vi "ImagingCore(HS).vi"(5 "BioMAP file path":path=path "", 7 "Params.":variant, 8 "error in (no error)":errorcluster, 9 "Dynamic Params queue":refnum<queue>, 10 "Quit_UserEvent":refnum<user-event>, 11 "ControlQueueRef":variant) -> (0 "error out":errorcluster, 2 "Output":variant)   [LabVIEW 2014]
uses:
  Apps_static/ScanParams_SingleLine.ctl
  Files/BinaryHeader.ctl
  ControlDef/QueueRefs.ctl
  ControlDef/LaserCtrl_Method.ctl
  ControlDef/States-AToF.ctl
  <instrlib>/GenericDAQ/VI/GenericDAQ_Ctrl_Queue.ctl
  <instrlib>/GenericDAQ/VI/GenericDAQ_State.ctl
  <instrlib>/ESP300/Public/Data/ESP300_State.ctl
  <instrlib>/DG535/Command/DG535_States.ctl
  Hardware/BNC(QuantumComposers)/BNC_States.ctl
  Hardware/FemtoLaser(Legacy)/Laser_Status.ctl
  Hardware/DAQmx(Legacy)/DAQmx_Status.ctl
  ControlDef/Signal.ctl
  ProcessMethods/SignalAverager/ProcessStates.ctl
  Files/WriterState.ctl
  <instrlib>/GenericDAQ/VI/GenericDAQ_Signal.ctl
  Hardware/EPM2000(Legacy)/EPM2K_Status.ctl
  ControlDef/SampleRateSelector.ctl
  ImagingMS/DirectImaging_State.ctl
  ImagingMS/Imaging_Params.ctl
  ProcessMethods/BioMapConversion/BioMAPWriterCoreParams.ctl
  ProcessMethods/Binning/BinType.ctl
  <vilib>/Utility/error.llb/DialogType.ctl
  <vilib>/Utility/miscctls.llb/LVRowAndColumnTypeDef.ctl
  <vilib>/picture/picture.llb/imagedata.ctl
  <vilib>/regexp/Match Regular Expression.xnode
  <instrlib>/ESP300/ESP300.lvlib
  <instrlib>/DG535/SRS_DG535_Lib.lvlib
  <userlib>/Utility/ErrorLog_lib.lvlib
  <instrlib>/GenericDAQ/GenericDAQ.lvlib
panel:
  out "Numeric":i32
  out "elements":i32[](array[numeric])
  out "segment #":i32
  out "EOL interval":dbl format="%#.6f"
  out "discarded ct":i32
  out "Flag":T1(ring)
  out "line time":dbl
  out "EOL time":dbl format="%_19f"
  out "line start time":dbl format="%_19f"
  in  "Full Image":bool
  out "flushing time":dbl
  in  "Contrast":cluster{dbl, dbl}(slide)={0.0, 255.0} scale=0.0..255.0
  in  "MaxiMass":dbl=300.0 format="%#_13g"
  in  "Binning":bool
  out "Information":string
  in  "AutoScaleZ":bool
  in  "SaveImage":bool
  in  "Color Scheme":T2(ring)=enum."Rainbow"
  out "#SOL":i32
  out "#EOL":i32
  out "remaining lines":i32
  out "State":T3(ring)
  out "Line# (Y_Img)":i32
  in  "Cancel":bool
  in  "Close/Quit":bool
  in  "Peaks of Interest (32 max)":string[][](table)=[["300", "300"], ["58", ".45"], ["92", ".45"], ["114", ".45"]]
  out "# average":i32
  in  "Start":bool
  out "ImagePreview":dbl[][](graph)
  in  "PeakOI #":i32 min=0 step=1
  out "MS (Raw)":cluster{"m/z_Array":dbl[], sgl[]}(graph)
  out "Iteration":i32
  out "Export File Path":path caption="Filename"
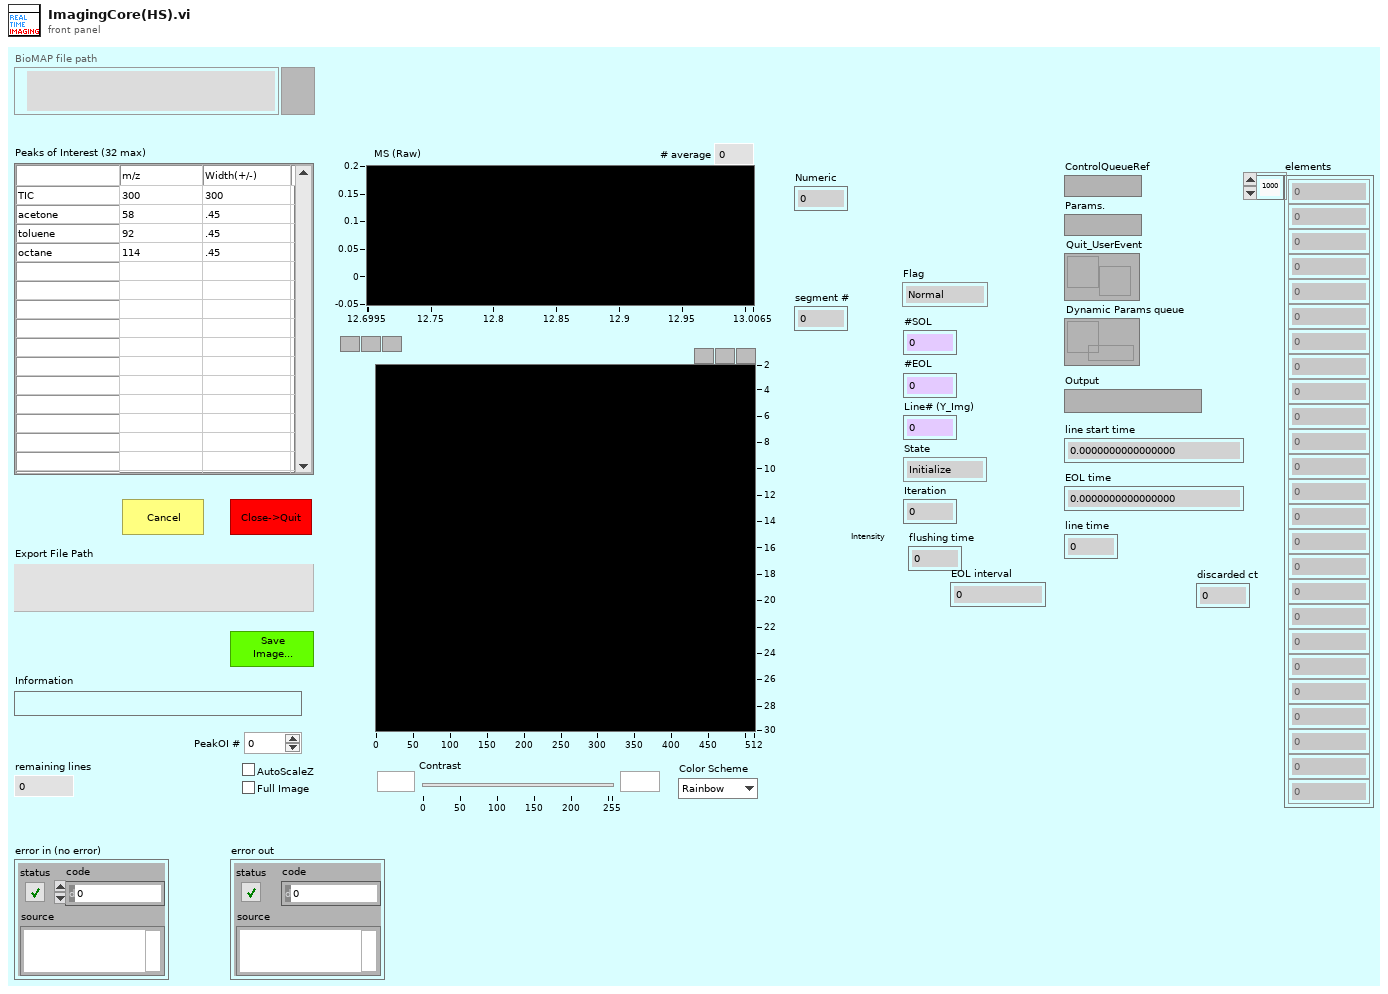
[diagram p1: front panel]
types:
  T1 = enum16{"Normal", "LineStart", "LineEnd", "FrameStart", "FrameEnd", "Reserved1", "Reserved2"}
  T2 = enum16{"Greyscale", "Rainbow", "Jet", "Rainbow_Wh", "Banded", "Seis", "InvertSeis", "Jaisnd", "TBD1"}
  T3 = enum16{"Initialize", "Open", "PrepScanParams", "WaitData", "Flush", "ScanResult", "CheckEndCondition", "Close", "Quit", "Refresh_Image", "Refresh_Profile", "Refresh_Spectra", "Refresh_RawSpectrum", "SaveMiddleFile", "Save_Image", "SetPeakOI"}
  T4 = enum8{"Enabled", "Disabled", "Disabled and Grayed Out"}
  T5 = typedef "QueueRefs.ctl" = cluster{"LaserCtrlMethod":T6, "Apps":refnum<queue>, "MainDAQCoreQueue":refnum<queue>, "Micos":refnum<queue>, "ESP300":refnum<queue>, "SMC100":refnum<queue>, "SRS DG535":refnum<queue>, "BNC":refnum<queue>, "SDG_ii":refnum<queue>, "NI-USB_DAQmx":refnum<queue>, "ProcCore_CtrlQueue":refnum<queue>, "WriterCtrl":refnum<queue>, "WriterSIG":refnum<queue>, "Feedback":refnum<queue>, "EPM2000":refnum<queue>, "InfoRef":refnum<vi>, "AppsLock":T7, "ProcCore_SignalBuffer":refnum<queue>}
  T6 = typedef "LaserCtrl_Method.ctl" = enum16{"SRS_DG535", "BNC", "SDG_II", "GenericDAQ_Sim"}
  T7 = typedef "Semaphore RefNum" = refnum<k1>
  T8 = typedef "BioMAPWriterCoreParams.ctl" = cluster{"File Header":T9, "mzCali.":dbl[], "m/z_Array":dbl[], "SampleRate":T10, "TrigDelay":dbl, "file refnum":refnum<file>, "file path":path, "PeakOI":cluster{"m/z":dbl, "Width(+/-)":dbl}[], "Binning":cluster{"Enable":bool, "BinType":T11, "BinWidth":dbl, "Maximum":dbl, "Minimum":dbl}}
  T9 = typedef "BinaryHeader.ctl" = cluster{"Start Position":dbl[], "StepWidth":dbl[], "Dimension":i32[], "SpecLength":i32}
  T10 = typedef "SampleRateSelector.ctl" = dbl
  T11 = typedef "BinType.ctl" = enum16{"ByTime", "ByScreen", "ByMass", "ToUnitMass"}
  T12 = typedef "Imaging_Params.ctl" = cluster{"File Header":T9, "ScanSpeed":dbl, "HighSpeed":dbl, "SampleRate":T10, "Rep.Rate (Hz)":dbl, "TrigDelay":dbl, "mzCali":dbl[], "KeepStill(ms)":u32, "SaveRaw":bool, "MultiRec":bool}
  T13 = typedef "DirectImaging_State.ctl" = cluster{"State":enum16{"Initialize", "Open", "PrepScanParams", "WaitData", "Flush", "ScanResult", "CheckEndCondition", "Close", "Quit", "Refresh_Image", "Refresh_Profile", "Refresh_Spectra", "Refresh_RawSpectrum", "SaveMiddleFile", "Save_Image", "SetPeakOI"}, "Para.":variant}
  T14 = cluster{"Save?":bool, "File Header":T9, "Scan#":i32, "ControlRefs":T5, "HighSpeed":dbl, "ScanSpeed":dbl, "SampleRate":T10, "mzCali.":dbl[], "TrigDelay":dbl, "InfoBarRef.":refnum<vi>, "MultiRec Mode":bool, "EOL_cts":i32, "SOL_cts":i32}
  T15 = typedef "LVRowAndColumnTypeDef.ctl" = cluster{"Row":i32, "Column":i32}
  T16 = typedef "DialogType.ctl" = u16
  T17 = typedef "GenericDAQ.lvlib/GenericDAQ_Signal.ctl" = cluster{"tickcount":u32, "Signal":sgl[], "SecondaryData":dbl[], "Flag":enum16{"Normal", "LineStart", "LineEnd", "FrameStart", "FrameEnd", "Reserved1", "Reserved2"}, "Segment#":i32}
  T18 = enum16{"open", "replace", "create", "open or create", "replace or create", "replace or create with confirmation"}
  T19 = typedef "Signal.ctl" = cluster{"Command":T20, "Params":variant}
  T20 = typedef "ProcessStates.ctl" = enum16{"Initialize", "Normal", "Display", "Write2Buffer", "CalcMzArray", "StartSave", "StopSave", "ConfigChanged", "EndOfLine", "SetFilterParams", "SetGraphsEnable", "SetAcquisitionParams", "ChangeDisplayIncrement", "ChangeRepRate", "SetWriterRef", "Quit", "StartOfLine"}
  T21 = typedef "GenericDAQ.lvlib/GenericDAQ_Ctrl_Queue.ctl" = cluster{"GenericDAQ State":T22, "Variant":variant}
  T22 = typedef "GenericDAQ.lvlib/GenericDAQ_State.ctl" = enum16{"Enumerate", "Open", "Close", "CloseAll", "Reset", "Quit", "==Settings==", "SetAcquisition_", "SetChannels_", "SetTrigger_", "SetAnalogTrigDetector_", "SetSegment#_", "SetAll_AcquChTrig_", "fConfigurate", "fStart", "GetStatus", "_WaitForDone/Idle", "_GetData", "GetAcquisition", "GetChannels", "GetTrigger", "GetAll_AcquChTrig", "Abort", "==Messaging==", "_PushDataOut", "GetStat_", "GetConfig_", "==ModeSetup==", "SetSignalBuffer_", "SetMode_", "SetSecondaryDataRef._", "SetDynamicBuffer_", "==AnalogOut==", "GetChannelCount_AO", "fStart_AO", "SetChEnable_AO", "SetConfig_AO", "SetFuncData_AO", "SetOffset_AO_", "SetMasterNode_AO", "SetStates_AO", "SetSymetry_AO", "SetTriggerSource_AO", "==Trigger==", "ManualTrigger", "===Sync===", "LineStart", "LineEnd", "FrameStart", "FrameEnd", "EOL_PassThrough", "SOL_PassThrough"}
  T23 = typedef "ScanParams_SingleLine.ctl" = cluster{"Line Start":dbl[], "Line End":dbl[], "HighSpeed":dbl, "ScanSpeed":dbl, "KeepStill(ms)":u32, "SecendaryParams":variant}
  T24 = typedef "imagedata.ctl" = cluster{"image type":i32, "image depth":i32, "image":u8[], "mask":u8[], "colors":u32[], "Rectangle":cluster{"left":i16, "top":i16, "right":i16, "bottom":i16}}
  T25 = cluster{"Rows Per Strip":i32, "Photometric":i32, "Compression Type":i32}
  T26 = cluster{"queue out":refnum<queue>, "queue out":refnum<queue>}
  T27 = typedef "IMAQ Image.ctl" = refnum<image>
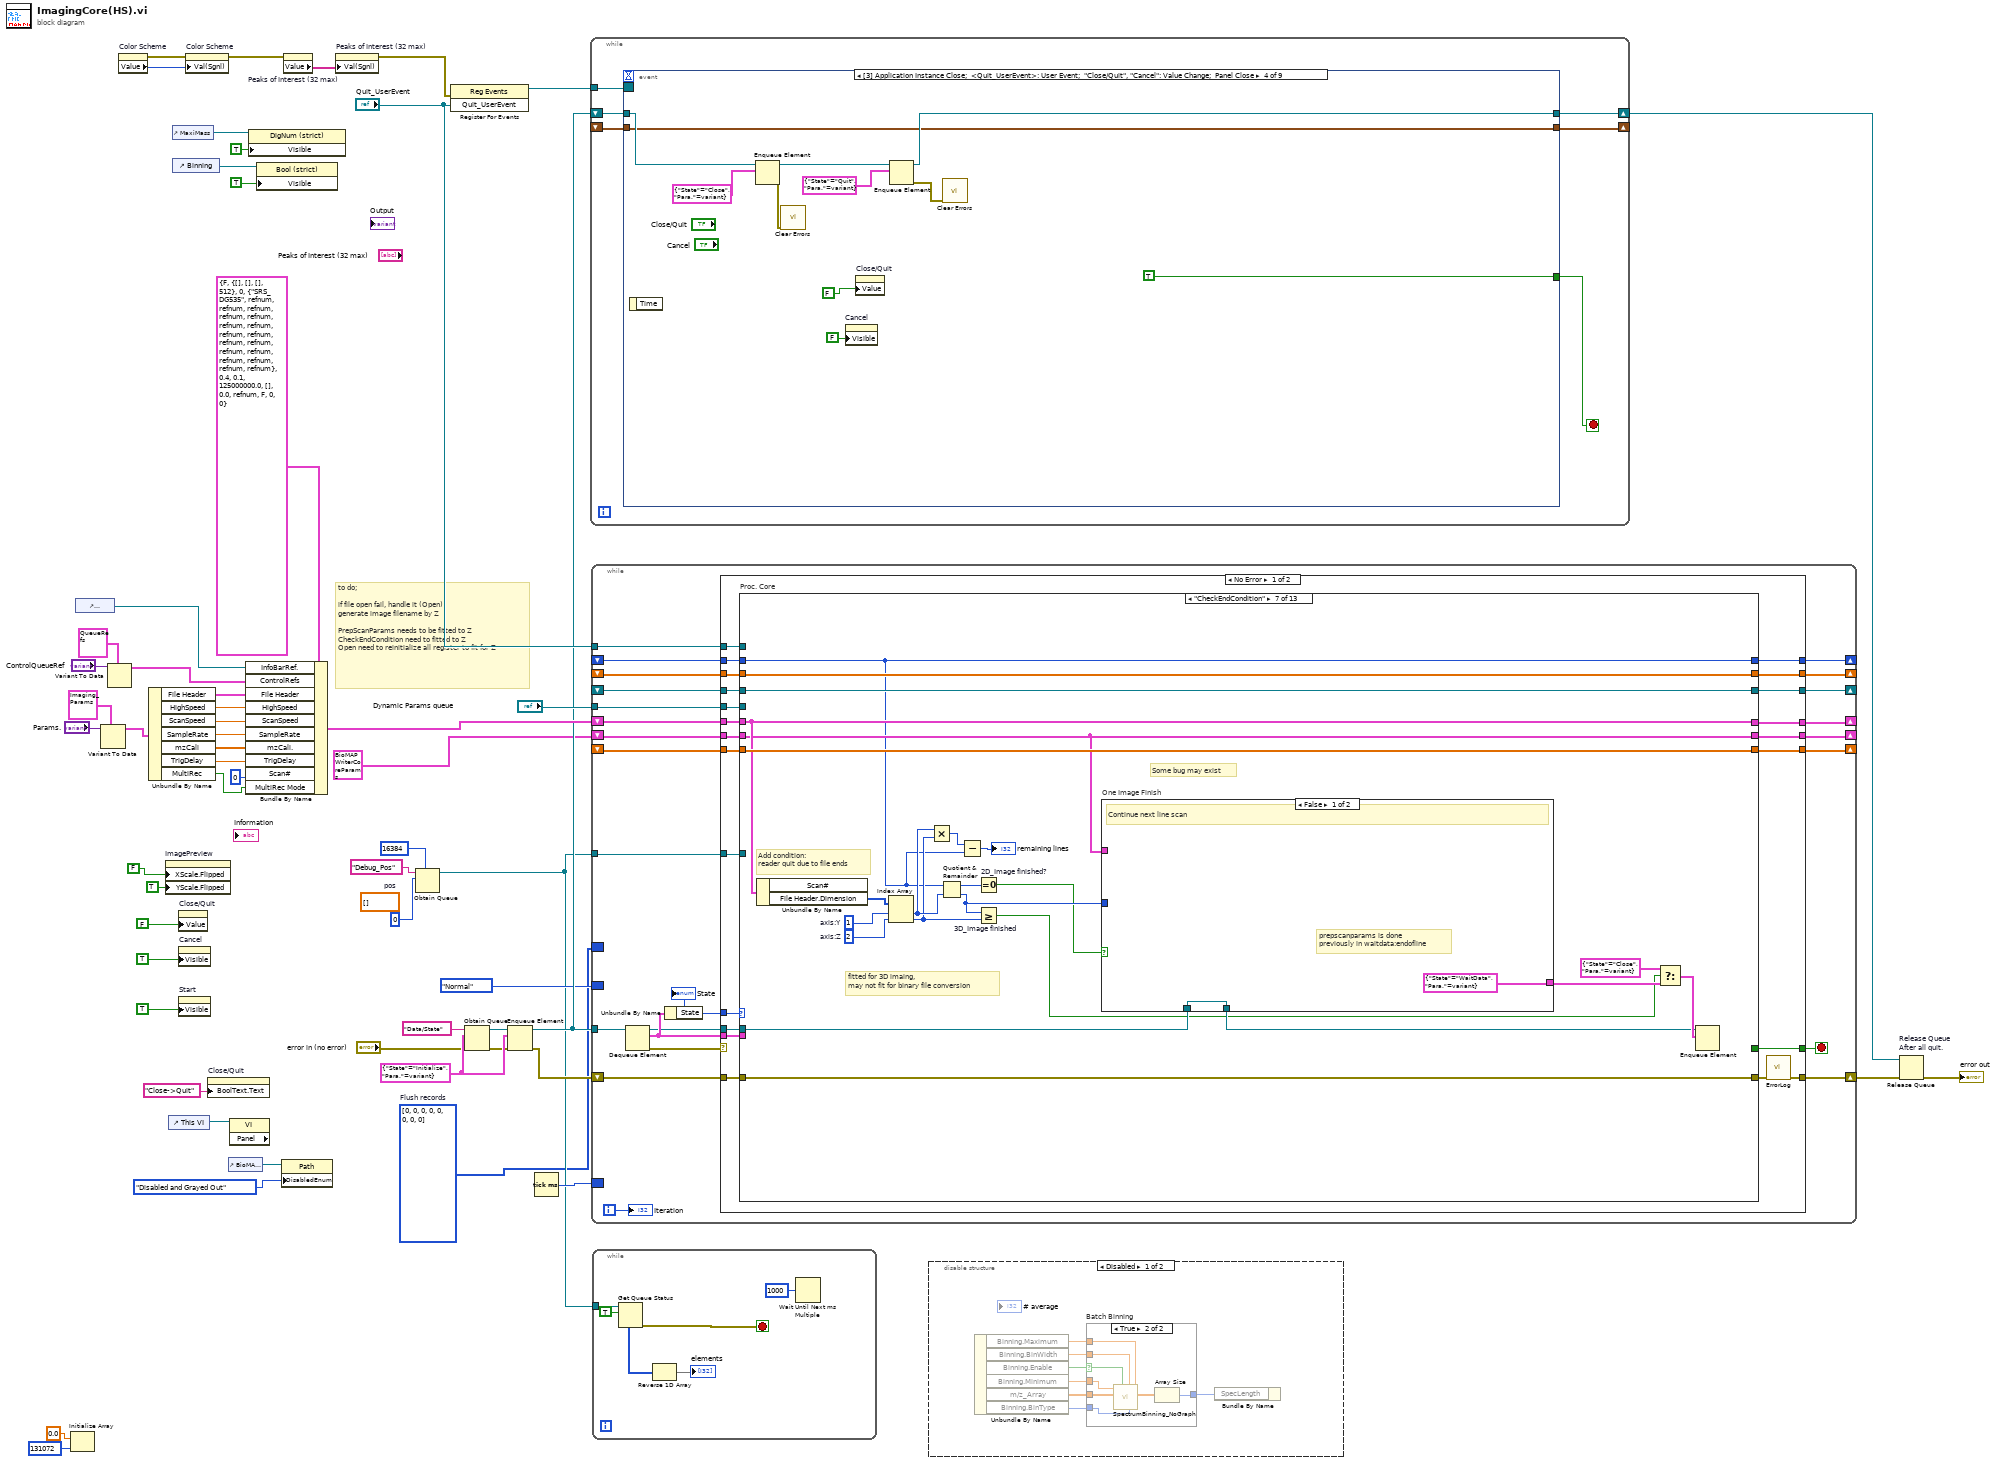
[diagram p0: block diagram]
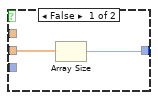
[diagram p2: hidden frame]
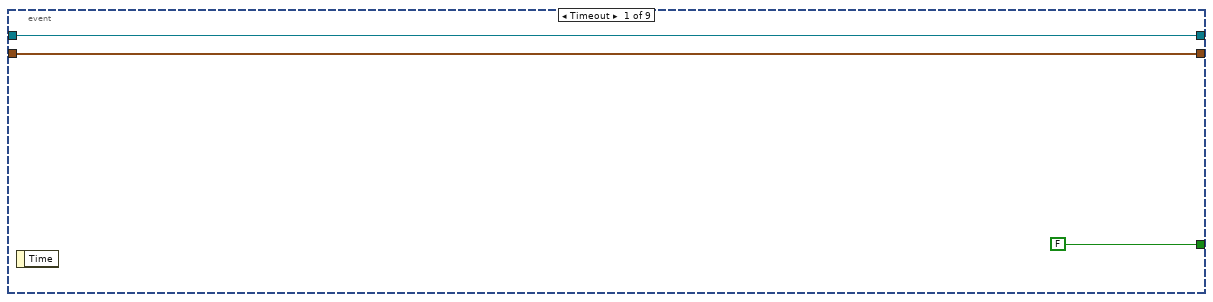
[diagram p4: hidden frame]
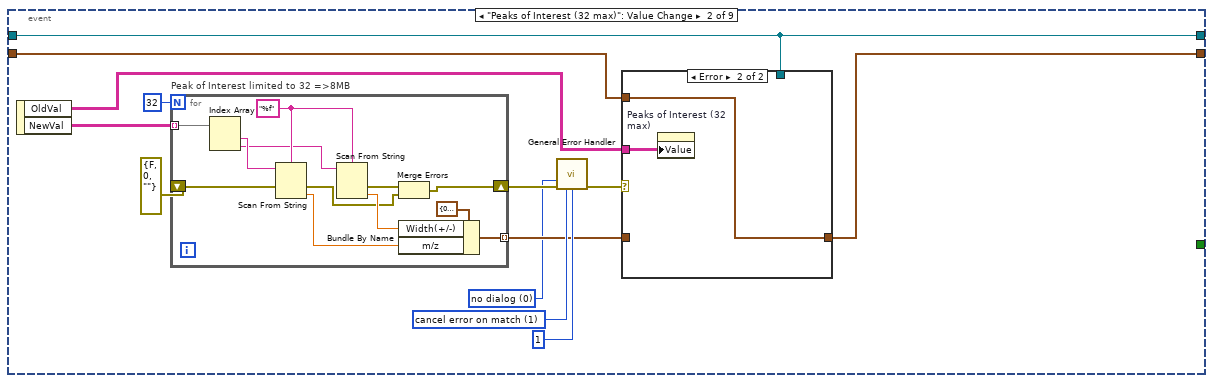
[diagram p5: hidden frame]
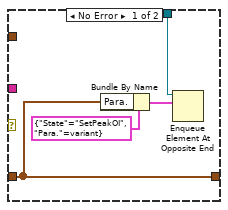
[diagram p6: hidden frame]
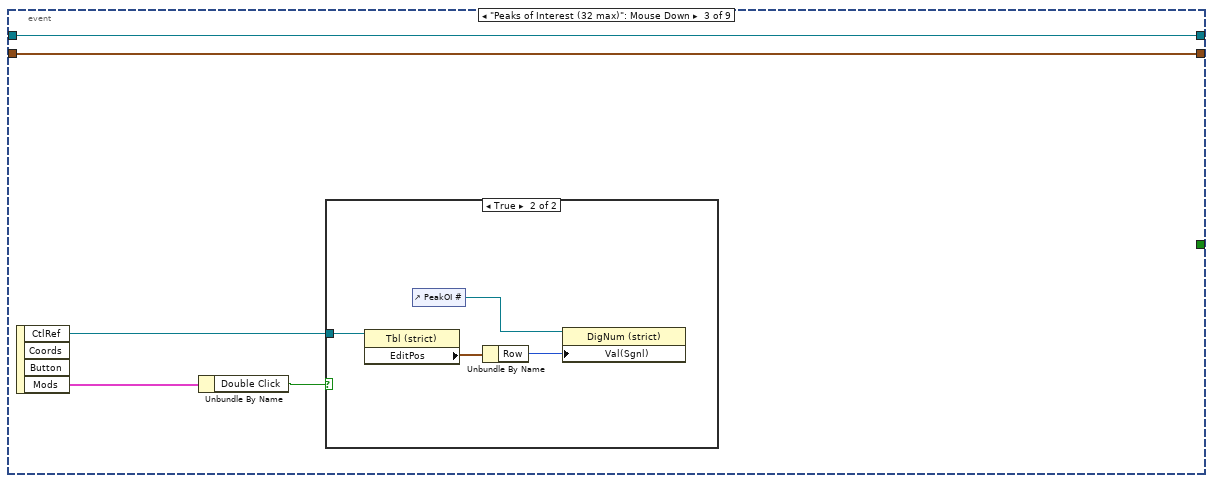
[diagram p7: hidden frame]
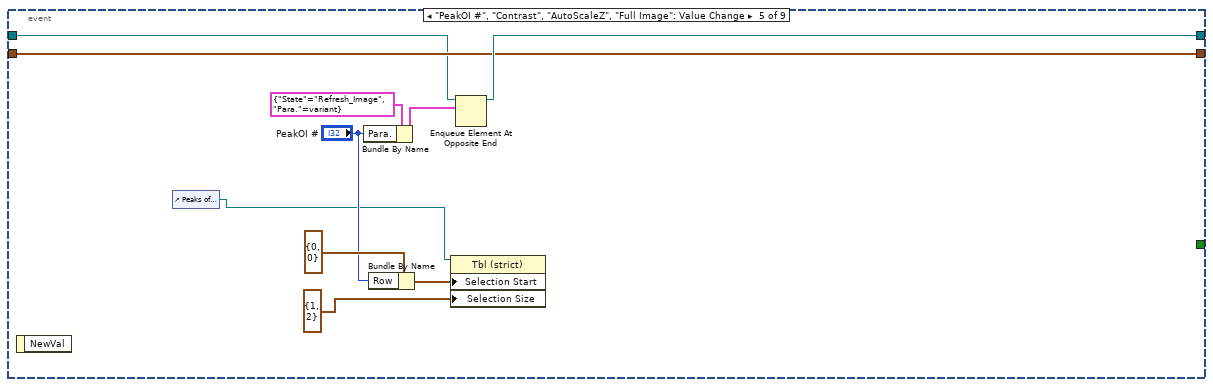
[diagram p9: hidden frame]
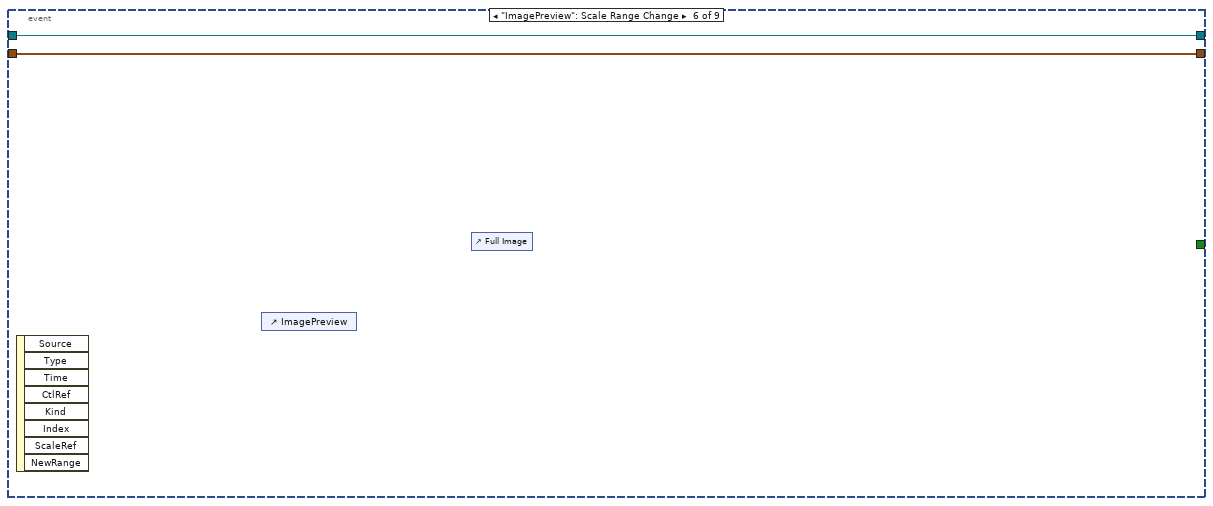
[diagram p10: hidden frame]
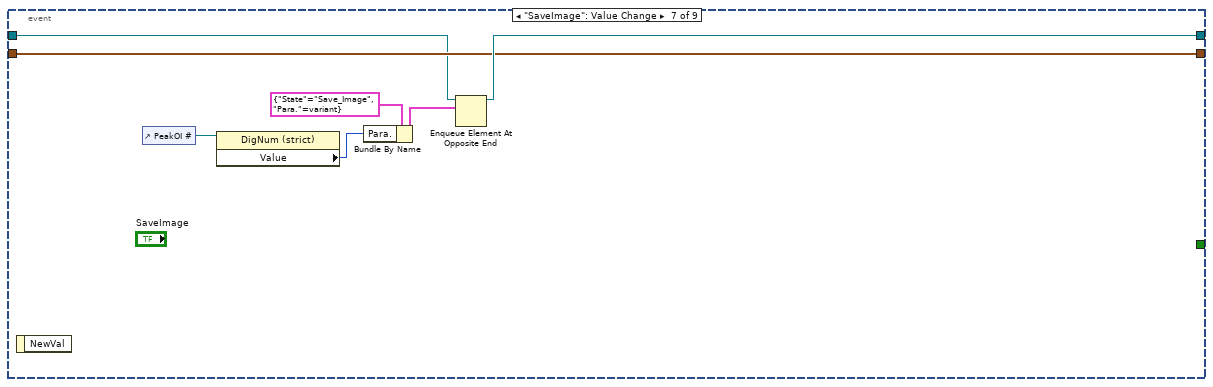
[diagram p11: hidden frame]
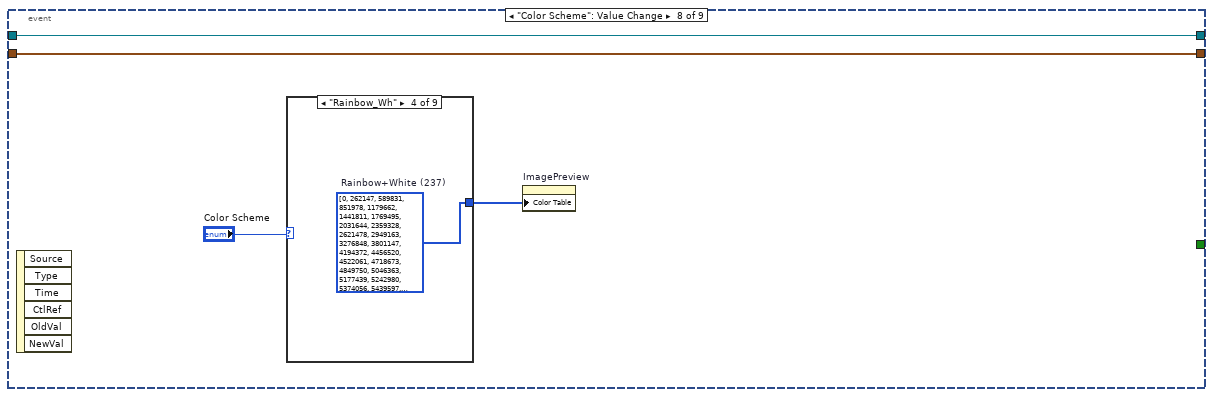
[diagram p12: hidden frame]
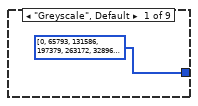
[diagram p13: hidden frame]
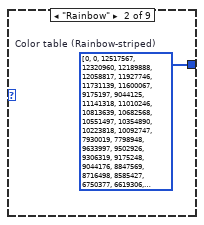
[diagram p14: hidden frame]
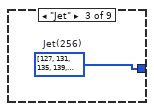
[diagram p15: hidden frame]
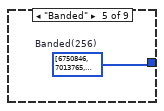
[diagram p16: hidden frame]
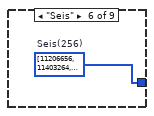
[diagram p17: hidden frame]
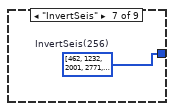
[diagram p18: hidden frame]
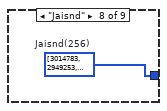
[diagram p19: hidden frame]
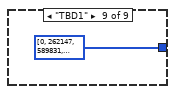
[diagram p20: hidden frame]
diagram:
  w2 = i32[] [0, 0, 0, 0, 0, 0, 0, 0]  # Flush records
  (unwired) dbl[] []  # pos
  w50 = T13 {"State"=enum."Initialize", "Para."=variant}
  # "to do;\n\nif file open fail, handle it (Open)\ngenerate image filename by Z\n\nPrepScanParams needs to be fitted to Z\nCheckEndCondition need to fitted to Z\nOpen need to reinitialize all register to fit for Z"
  n1 = Initialize Array(sgl 0.0 ("element"), 131072 ("dimension size")) -> ()  [unwired: 1 out]
  n2 = control-ref of="Information"() -> (w19:refnum<vi>)
  n3 = Variant To Data(type=T12 {"File Header"={"Start Position"=[], "StepWidth"=[], "Dimension"=[], "SpecLength"=0}, "ScanSpeed"=0.0, "HighSpeed"=0.0, "SampleRate"=0.0, "Rep.Rate (Hz)"=0.0, "TrigDelay"=0.0, "mzCali"=[], "KeepStill(ms)"=0, "SaveRaw"=FALSE, "MultiRec"=FALSE} ("BeamProfiling_Params"), Variant="Params.") -> (data=w45:T12)  [unwired: 1 in, 1 out]
  n4 = Variant To Data(type=T5 {"LaserCtrlMethod"=enum."SRS_DG535", "Apps"=refnum, "MainDAQCoreQueue"=refnum, "Micos"=refnum, "ESP300"=refnum, "SMC100"=refnum, "SRS DG535"=refnum, "BNC"=refnum, "SDG_ii"=refnum, "NI-USB_DAQmx"=refnum, "ProcCore_CtrlQueue"=refnum, "WriterCtrl"=refnum, "WriterSIG"=refnum, "Feedback"=refnum, "EPM2000"=refnum, "InfoRef"=refnum, "AppsLock"=refnum, "ProcCore_SignalBuffer"=refnum} ("ControlRefs"), Variant="ControlQueueRef") -> (data=w27:T5)  [unwired: 1 in, 1 out]
  n5 = property on="Color Scheme" class="Enum (strict)"() -> (error out=w16:errorcluster, "Value"=w17:T2)  [unwired: 2 in, 1 out]
  n6 = Unbundle By Name(w45) -> ("File Header"=w44:T9, "HighSpeed"=w43:dbl, "ScanSpeed"=w42:dbl, "SampleRate"=w40:T10, "mzCali"=w32:dbl[], "TrigDelay"=w31:dbl, "MultiRec"=w3:bool)
  n7 = property on="ImagePreview" class="IntGraph (strict)"("XScale.Flipped"=FALSE, "YScale.Flipped"=TRUE ("Y Scale.Flipped")) -> ()  [unwired: 2 in, 2 out]
  n8 = control-ref of="This VI"() -> (w30:refnum<vi>)
  n9 = control-ref of="MaxiMass"() -> (w13:refnum<vi>)
  n10 = control-ref of="Binning"() -> (w10:refnum<vi>)
  n11 = property on="Close/Quit" class="Bool (strict)"("Value"=FALSE) -> ()  [unwired: 2 in, 2 out]
  n12 = property on="Cancel" class="Bool"("Visible"=TRUE) -> ()  [unwired: 2 in, 2 out]
  n13 = property on="Start" class="Bool"("Visible"=TRUE) -> ()  [unwired: 2 in, 2 out]
  n14 = property on="Color Scheme" class="Enum (strict)"(error in=w16, "Val(Sgnl)"=w17) -> (error out=w14:errorcluster)  [unwired: 1 in, 1 out]
  n15 = property on="Close/Quit" class="Bool (strict)"("BoolText.Text"="Close->Quit" ("Boolean Text.Text")) -> ()  [unwired: 2 in, 2 out]
  n16 = control-ref of="BioMAP file path"() -> (w26:refnum<vi>)
  n17 = property class="VI" props=["Panel"](reference=w30) -> ()  [unwired: 1 in, 3 out]
  n18 = Bundle By Name(cluster=T14 {"Save?"=FALSE, "File Header"={"Start Position"=[], "StepWidth"=[], "Dimension"=[], "SpecLength"=512}, "Scan#"=0, "ControlRefs"={"LaserCtrlMethod"=enum."SRS_DG535", "Apps"=refnum, "MainDAQCoreQueue"=refnum, "Micos"=refnum, "ESP300"=refnum, "SMC100"=refnum, "SRS DG535"=refnum, "BNC"=refnum, "SDG_ii"=refnum, "NI-USB_DAQmx"=refnum, "ProcCore_CtrlQueue"=refnum, "WriterCtrl"=refnum, "WriterSIG"=refnum, "Feedback"=refnum, "EPM2000"=refnum, "InfoRef"=refnum, "AppsLock"=refnum, "ProcCore_SignalBuffer"=refnum}, "HighSpeed"=0.4, "ScanSpeed"=0.1, "SampleRate"=125000000.0, "mzCali."=[], "TrigDelay"=0.0, "InfoBarRef."=refnum, "MultiRec Mode"=FALSE, "EOL_cts"=0, "SOL_cts"=0} ("output cluster"), "InfoBarRef."=w19, "ControlRefs"=w27, "File Header"=w44, "HighSpeed"=w43, "ScanSpeed"=w42, "SampleRate"=w40, "mzCali."=w32, "TrigDelay"=w31, "Scan#"=0, "MultiRec Mode"=w3) -> (w54:T14)
  n19 = property class="DigNum (strict)"(reference=w13, "Visible"=TRUE) -> ()  [unwired: 1 in, 2 out]
  n20 = property class="Bool (strict)"(reference=w10, "Visible"=TRUE) -> ()  [unwired: 1 in, 2 out]
  n21 = property class="Path"(reference=w26, "DisabledEnum"=T4."Disabled and Grayed Out" ("Disabled")) -> ()  [unwired: 1 in, 2 out]
  n22 = property on="Peaks of Interest (32 max)" class="Tbl (strict)"(error in=w14) -> ("Value"=w21:string[][])  [unwired: 1 in, 2 out]
  n23 = property on="Peaks of Interest (32 max)" class="Tbl (strict)"("Val(Sgnl)"=w21) -> (error out=w15:errorcluster)  [unwired: 2 in, 1 out]
  n24 = Obtain Queue(max queue size (-1, unlimited)=16384, name (unnamed)="Debug_Pos", element data type=0) -> (queue out=w4:refnum<queue>)  [unwired: 2 in, 2 out]
  n25 = register-events(error in=w15, "Quit_UserEvent") -> (reference out=w55:refnum<event-registration>)  [unwired: 1 in, 1 out]
  n26 = Obtain Queue(name (unnamed)="Data/State", element data type=w50, error in (no error)="error in (no error)") -> (queue out=w51:refnum<queue>, error out=w49:errorcluster)  [unwired: 2 in, 1 out]
  n27 = Enqueue Element(queue=w51, element=w50, error in (no error)=w49) -> (queue out=w47:refnum<queue>, error out=w39:errorcluster)  [unwired: 1 in, 1 out]
  n28 = Tick Count (ms)() -> (millisecond timer value=w38:u32)
  n29 = while {
    tunnel: w55 -> [w62]
    shift-right: [w61] -> w33
    shift-left: w47 -> [w64]
    shift-right: [w60] -> _
    shift-left: _ -> [w59]
    stop <- w63 stop-if-true
    n30 = event shown="[3] Application Instance Close;  <Quit_UserEvent>: User Event;  \"Close/Quit\", \"Cancel\": Value Change;  Panel Close" {
      selector: w62 -> [_ _ _ _ _ _ _ _ _]
      dyn-events: _ -> [_ _ _ _ _ _ _ _ _]
      timeout: _ -> [_ _ _ _ _ _ _ _ _]
      tunnel: w64 -> [w66 w68 w103 w115 w124 w130 w133 w141 w159]
      tunnel: [FALSE _ _ TRUE _ _ _ _ _] -> w63
      tunnel: [w66 w68 w103 w111 w126 w130 w135 w141 w154] -> w61
      tunnel: [w65 w73 w99 w110 w125 w129 w134 w138 w156] -> w60
      tunnel: w59 -> [w65 w71 w99 w110 w125 w129 w134 w138 w156]
      event Timeout {
        n31 = event-data() -> ()  [unwired: 1 in, 1 out]
      }
      event "Peaks of Interest (32 max)": Value Change {
        w69 = T16 0 items=["no dialog", "OK message", "continue or stop message", "OK message + warnings", "continue/stop + warnings"] ("type of dialog (OK msg:1)")
        w74 = 1 items=["no exception", "cancel error on match", "set error on match"] ("[exception action] (none:0)")
        n32 = event-data() -> ("OldVal"=w79:string[][], "NewVal"=w80:string[][])  [unwired: 1 in]
        n33 = for "Peak of Interest limited to 32 =>8MB" {
          N: 32 -> [_]
          tunnel: w80 -> [w92] mode=indexing
          shift-right: [w84] -> w75
          shift-left: errorcluster {"status"=FALSE, "code"=0, "source"=""} ("error IO") -> [w86]
          tunnel: [w85] -> w72 mode=indexing
          w91 = "%f" ("format string")
          n34 = Index Array(array=w92) -> (element #1=w82:string, element #2=w81:string)  [unwired: 2 in]
          n35 = Scan From String(format string=w91, input string=w82, error in=w86) -> (error out=w83:errorcluster, output 1=w88:dbl)  [unwired: 2 in, 2 out]
          n36 = Scan From String(format string=w91, input string=w81) -> (error out=w87:errorcluster, output 1=w89:dbl)  [unwired: 3 in, 2 out]
          n37 = Merge Errors(w87, w83) -> (w84:errorcluster)
          n38 = Bundle By Name(cluster=cluster{"m/z":dbl, "Width(+/-)":dbl} {"m/z"=0.0, "Width(+/-)"=0.0} ("Peak-Of-Interest"), "Width(+/-)"=w89, "m/z"=w88) -> (w85:cluster{"m/z":dbl, "Width(+/-)":dbl})
        }
        n39 = call <vilib>:"General Error Handler.vi"("type of dialog (OK msg:1)"=w69, "error in (no error)"=w75, "[exception action] (none:0)"=w74, "[exception code]"=1) -> ("error out"=w76:errorcluster)  [unwired: 7 in, 4 out]
        n40 = case shown="Error" w76 {
          tunnel: w79 -> [_ w98]
          tunnel: [w94 w97] -> w73
          tunnel: w72 -> [w94 _]
          tunnel: w71 -> [_ w97]
          tunnel: w68 -> [w93 _]
          frame No Error {
            n41 = Bundle By Name(cluster=T13 {"State"=enum."SetPeakOI", "Para."=variant} ("element"), "Para."=w94) -> (w95:T13)
            n42 = Enqueue Element At Opposite End(queue=w93, element=w95) -> ()  [unwired: 2 in, 3 out]
          }
          frame Error {
            n43 = property on="Peaks of Interest (32 max)" class="Tbl (strict)"("Value"=w98) -> ()  [unwired: 2 in, 2 out]
          }
        }
      }
      event "Peaks of Interest (32 max)": Mouse Down {
        n44 = event-data() -> ("CtlRef"=w100:refnum<vi>, "Mods"=w101:cluster{"Double Click":bool, "Menu Key":bool})  [unwired: 1 in, 2 out]
        n45 = Unbundle By Name(w101) -> ("Double Click"=w102:bool)
        n46 = case shown="True" w102 {
          tunnel: w100 -> [_ w106]
          frame False {
          }
          frame True {
            n47 = property class="Tbl (strict)"(reference=w106) -> ("EditPos"=w107:T15)  [unwired: 1 in, 2 out]
            n48 = control-ref of="PeakOI #"() -> (w104:refnum<vi>)
            n49 = Unbundle By Name(w107) -> ("Row"=w105:i32)
            n50 = property class="DigNum (strict)"(reference=w104, "Val(Sgnl)"=w105) -> ()  [unwired: 1 in, 2 out]
          }
        }
      }
      event Application Instance Close; User Event; "Close/Quit", "Cancel": Value Change; Panel Close {
        n51 = event-data() -> ()  [unwired: 1 in, 1 out]
        n52 = Enqueue Element(queue=w115, element=T13 {"State"=enum."Close", "Para."=variant}) -> (queue out=w116:refnum<queue>, error out=w114:errorcluster)  [unwired: 2 in, 1 out]
        n53 = call <vilib>:"Clear Errors.vi"("error in (no error)"=w114) -> ()  [unwired: 5 in, 2 out]
        n54 = property on="Cancel" class="Bool"("Visible"=FALSE) -> ()  [unwired: 2 in, 2 out]
        n55 = property on="Close/Quit" class="Bool (strict)"("Value"=FALSE) -> ()  [unwired: 2 in, 2 out]
        n56 = Enqueue Element(queue=w116, element=T13 {"State"=enum."Quit", "Para."=variant}) -> (queue out=w111:refnum<queue>, error out=w117:errorcluster)  [unwired: 2 in, 1 out]
        n57 = call <vilib>:"Clear Errors.vi"("error in (no error)"=w117) -> ()  [unwired: 5 in, 2 out]
      }
      event "PeakOI #", "Contrast", "AutoScaleZ", "Full Image": Value Change {
        n58 = event-data() -> ()  [unwired: 1 in, 1 out]
        n59 = control-ref of="Peaks of Interest (32 max)"() -> (w119:refnum<vi>)
        n60 = Bundle By Name(cluster=T13 {"State"=enum."Refresh_Image", "Para."=variant} ("element"), "Para."="PeakOI #") -> (w127:T13)
        n61 = Bundle By Name(cluster=T15 {"Row"=0, "Column"=0} ("Selection Start"), "Row"="PeakOI #") -> (w122:T15)
        n62 = property on="Property Node" class="Tbl (strict)"(reference=w119, "Selection Start"=w122, "Selection Size"=T15 {"Row"=1, "Column"=2}) -> ()  [unwired: 1 in, 2 out]
        n63 = Enqueue Element At Opposite End(queue=w124, element=w127) -> (queue out=w126:refnum<queue>)  [unwired: 2 in, 2 out]
      }
      event "ImagePreview": Scale Range Change {
        n64 = event-data() -> ()  [unwired: 1 in, 8 out]
        n65 = control-ref of="ImagePreview"() -> ()  [unwired: 1 out]
        n66 = control-ref of="Full Image"() -> ()  [unwired: 1 out]
      }
      event "SaveImage": Value Change {
        n67 = event-data() -> ()  [unwired: 1 in, 1 out]
        n68 = control-ref of="PeakOI #"() -> (w132:refnum<vi>)
        n69 = property class="DigNum (strict)"(reference=w132) -> ("Value"=w131:i32)  [unwired: 1 in, 2 out]
        n70 = Bundle By Name(cluster=T13 {"State"=enum."Save_Image", "Para."=variant} ("element"), "Para."=w131) -> (w136:T13)
        n71 = Enqueue Element At Opposite End(queue=w133, element=w136) -> (queue out=w135:refnum<queue>)  [unwired: 2 in, 2 out]
      }
      event "Color Scheme": Value Change {
        n72 = event-data() -> ()  [unwired: 1 in, 6 out]
        n73 = case shown="\"Rainbow_Wh\"" "Color Scheme" {
          tunnel: [u32[] [0, 65793, 131586, 197379, 263172, 328965, 394758, 460551, 526344, 592137, 657930, 723723, 789516, 855309, 921102, 986895, 1052688, 1118481, 1184274, 1250067, 1315860, 1381653, 1447446, 1513239, 1579032, 1644825, 1710618, 1776411, 1842204, 1907997, 1973790, 2039583, 2105376, 2171169, 2236962, 2302755, 2368548, 2434341, 2500134, 2565927, 2631720, 2697513, 2763306, 2829099, 2894892, 2960685, 3026478, 3092271, 3158064, 3223857, 3289650, 3355443, 3421236, 3487029, 3552822, 3618615, 3684408, 3750201, 3815994, 3881787, 3947580, 4013373, 4079166, 4144959, 4210752, 4276545, 4342338, 4408131, 4473924, 4539717, 4605510, 4671303, 4737096, 4802889, 4868682, 4934475, 5000268, 5066061, 5131854, 5197647, 5263440, 5329233, 5395026, 5460819, 5526612, 5592405, 5658198, 5723991, 5789784, 5855577, 5921370, 5987163, 6052956, 6118749, 6184542, 6250335, 6316128, 6381921, 6447714, 6513507, 6579300, 6645093, 6710886, 6776679, 6842472, 6908265, 6974058, 7039851, 7105644, 7171437, 7237230, 7303023, 7368816, 7434609, 7500402, 7566195, 7631988, 7697781, 7763574, 7829367, 7895160, 7960953, 8026746, 8092539, 8158332, 8224125, 8289918, 8355711, 8421504, 8487297, 8553090, 8618883, 8684676, 8750469, 8816262, 8882055, 8947848, 9013641, 9079434, 9145227, 9211020, 9276813, 9342606, 9408399, 9474192, 9539985, 9605778, 9671571, 9737364, 9803157, 9868950, 9934743, 10000536, 10066329, 10132122, 10197915, 10263708, 10329501, 10395294, 10461087, 10526880, 10592673, 10658466, 10724259, 10790052, 10855845, 10921638, 10987431, 11053224, 11119017, 11184810, 11250603, 11316396, 11382189, 11447982, 11513775, 11579568, 11645361, 11711154, 11776947, 11842740, 11908533, 11974326, 12040119, 12105912, 12171705, 12237498, 12303291, 12369084, 12434877, 12500670, 12566463, 12632256, 12698049, 12763842, 12829635, 12895428, 12961221, 13027014, 13092807, 13158600, 13224393, 13290186, 13355979, 13421772, 13487565, 13553358, 13619151, 13684944, 13750737, 13816530, 13882323, 13948116, 14013909, 14079702, 14145495, 14211288, 14277081, 14342874, 14408667, 14474460, 14540253, 14606046, 14671839, 14737632, 14803425, 14869218, 14935011, 15000804, 15066597, 15132390, 15198183, 15263976, 15329769, 15395562, 15461355, 15527148, 15592941, 15658734, 15724527, 15790320, 15856113, 15921906, 15987699, 16053492, 16119285, 16185078, 16250871, 16316664, 16382457, 16448250, 16514043, 16579836, 16645629, 16711422, 16777215] ("Array") w143 w144 w145 w146 w147 w148 w149 u32[] [0, 262147, 589831, 851978, 1179662, 1441811, 1769495, 2031644, 2359328, 2621478, 2949163, 3276848, 3801147, 4194372, 4456520, 4522061, 4718673, 4849750, 5046363, 5177439, 5242980, 5374056, 5439597, 5505142, 5636218, 5767300, 5636232, 5701773, 5701777, 5701782, 5570714, 5505183, 5505187, 5505192, 5177521, 5111990, 5046458, 4980927, 4587720, 4456652, 4325585, 3932374, 3801306, 3604703, 3014888, 2818284, 2621681, 2359541, 2162938, 1638655, 1048831, 786687, 262399, 255, 1279, 4351, 5631, 6655, 7679, 9983, 11007, 12031, 13311, 16383, 17407, 18687, 21759, 23039, 24063, 25087, 27391, 28415, 29439, 30719, 32767, 34815, 36095, 39167, 40447, 41471, 42495, 44799, 45823, 46847, 48127, 50175, 51199, 55551, 56575, 57855, 58879, 59903, 62207, 63231, 64255, 65535, 65526, 65522, 65518, 65505, 65496, 65492, 65483, 65479, 65475, 65471, 65467, 65458, 65454, 65450, 65437, 65432, 65424, 65415, 65411, 65407, 65403, 65394, 65390, 65386, 65382, 65369, 65364, 65360, 65356, 65343, 65339, 65335, 65326, 65322, 65318, 65305, 65301, 65296, 65292, 65288, 65280, 589568, 851712, 1441536, 1703680, 1965824, 2817792, 3079936, 3407616, 3669760, 4194048, 4456192, 4783872, 5046016, 5897984, 6160128, 6422272, 7274240, 7536384, 7864064, 8126208, 8650496, 8912640, 9240320, 9502464, 10092288, 10616576, 10878720, 11730688, 11992832, 12320512, 12582656, 13106944, 13369088, 13696768, 13958912, 14548736, 14810880, 15924992, 16187136, 16449280, 16776960, 16775680, 16773632, 16772608, 16771328, 16770304, 16768256, 16766976, 16765952, 16762624, 16760576, 16759552, 16757248, 16756224, 16755200, 16753920, 16752896, 16750848, 16749568, 16748544, 16745216, 16744192, 16742144, 16739840, 16738816, 16737792, 16736512, 16734464, 16733440, 16732160, 16731136, 16727808, 16726784, 16725760, 16724736, 16721408, 16720384, 16719104, 16717056, 16716032, 16714752, 16711680, 16711680, 16711680, 16711680, 16711680, 16711680, 16711680, 16711680, 16711680, 16711680, 16711680, 16711680, 16711680, 16711680, 16711680, 16711680, 16711680, 16711680, 15527148, 15592941, 15658734, 15724527, 15790320, 15856113, 15921906, 15987699, 16053492, 16119285, 16185078, 16250871, 16316664, 16382457, 16448250, 16514043, 16579836, 16645629, 16711422, 16777215] ("appended array")] -> w139
          frame "Greyscale", Default {
          }
          frame "Rainbow" {
            w143 = u32[] [0, 0, 12517567, 12320960, 12189888, 12058817, 11927746, 11731139, 11600067, 9175197, 9044125, 11141318, 11010246, 10813639, 10682568, 10551497, 10354890, 10223818, 10092747, 7930019, 7798948, 9633997, 9502926, 9306319, 9175248, 9044176, 8847569, 8716498, 8585427, 6750377, 6619306, 8126677, 7995606, 7798999, 7667927, 7536856, 7340249, 7209178, 7078106, 5505199, 5374128, 6619357, 6488285, 6291678, 6160607, 6029536, 5832929, 5701857, 5570786, 4325557, 4194486, 5112036, 4980965, 4784358, 4653287, 4522215, 4325608, 4194537, 4063466, 3080380, 3014844, 3604716, 3408109, 3277038, 3277038, 3145966, 3014895, 2818288, 2687217, 2556145, 1900738, 1769666, 2097396, 1900789, 1769717, 1638646, 1507575, 1310968, 1179896, 1048825, 721096, 590024, 590075, 393468, 262397, 131326, 255, 1791, 3327, 4863, 5068, 6348, 9471, 11007, 12543, 14079, 15615, 17151, 18687, 20223, 17612, 18636, 25087, 26623, 28159, 29695, 31231, 32767, 34303, 35839, 29900, 31180, 40447, 41983, 43775, 45311, 46847, 48383, 49919, 51455, 42444, 43724, 56063, 57599, 59135, 60671, 62207, 63743, 65535, 65528, 52418, 52413, 65510, 65504, 65498, 65492, 65486, 65480, 65474, 65468, 52369, 52364, 65449, 65443, 65437, 65431, 65425, 65419, 65413, 65407, 52321, 52316, 65389, 65383, 65377, 65371, 65364, 65358, 65352, 65346, 52272, 52267, 65328, 65322, 65316, 65310, 65304, 65298, 65292, 65286, 52224, 314368, 851712, 1244928, 1638144, 2031360, 2424576, 2817792, 3211008, 3604224, 3197952, 3525632, 4783872, 5177088, 5635840, 6029056, 6422272, 6815488, 7208704, 7601920, 6409216, 6736896, 6736896, 8781568, 9174784, 9568000, 9961216, 10354432, 10747648, 11206400, 11599616, 9554944, 9882624, 12779264, 13172480, 13565696, 13958912, 14352128, 14745344, 15138560, 15531776, 12766208, 13093888, 16776960, 16775170, 16773637, 16771847, 16770314, 16768780, 16766991, 16765457, 13411088, 13409810, 16760601, 16758812, 16757278, 16755745, 16753955, 16752422, 16750888, 16749099, 13398052, 13396774, 16744243, 16742704, 16741166, 16739884, 16738345, 16736807, 16735269, 16733730, 13385753, 13384728, 16729371, 16727833, 16726295, 16725012, 16723474, 16721936, 16720397, 16718859, 13373959, 13372677, 16714500, 16712962, 16777215]  # Color table (Rainbow-striped)
          }
          frame "Jet" {
            w144 = u32[] [127, 131, 135, 139, 143, 147, 151, 155, 159, 163, 167, 171, 175, 179, 183, 187, 191, 195, 199, 203, 207, 211, 215, 219, 223, 227, 231, 235, 239, 243, 247, 251, 255, 1279, 2303, 3327, 4351, 5375, 6399, 7423, 8447, 9471, 10495, 11519, 12543, 13567, 14591, 15615, 16639, 17663, 18687, 19711, 20735, 21759, 22783, 23807, 24831, 25855, 26879, 27903, 28927, 29951, 30975, 31999, 33023, 34047, 35071, 36095, 37119, 38143, 39167, 40191, 41215, 42239, 43263, 44287, 45311, 46335, 47359, 48383, 49407, 50431, 51455, 52479, 53503, 54527, 55551, 56575, 57599, 58623, 59647, 60671, 61695, 62719, 63743, 64767, 131069, 393209, 655349, 917489, 1179629, 1441769, 1703909, 1966049, 2228189, 2490329, 2752469, 3014609, 3276749, 3538889, 3801029, 4063169, 4325309, 4587449, 4849589, 5111729, 5373869, 5636009, 5898149, 6160289, 6422429, 6684569, 6946709, 7208849, 7470989, 7733129, 7995269, 8257409, 8519549, 8781689, 9043829, 9305969, 9568109, 9830249, 10092389, 10354529, 10616669, 10878809, 11140949, 11403089, 11665229, 11927369, 12189509, 12451649, 12713789, 12975929, 13238069, 13500209, 13762349, 14024489, 14286629, 14548769, 14810909, 15073049, 15335189, 15597329, 15859469, 16121609, 16383749, 16645889, 16776192, 16775168, 16774144, 16773120, 16772096, 16771072, 16770048, 16769024, 16768000, 16766976, 16765952, 16764928, 16763904, 16762880, 16761856, 16760832, 16759808, 16758784, 16757760, 16756736, 16755712, 16754688, 16753664, 16752640, 16751616, 16750592, 16749568, 16748544, 16747520, 16746496, 16745472, 16744448, 16743424, 16742400, 16741376, 16740352, 16739328, 16738304, 16737280, 16736256, 16735232, 16734208, 16733184, 16732160, 16731136, 16730112, 16729088, 16728064, 16727040, 16726016, 16724992, 16723968, 16722944, 16721920, 16720896, 16719872, 16718848, 16717824, 16716800, 16715776, 16714752, 16713728, 16712704, 16711680, 16449536, 16187392, 15925248, 15663104, 15400960, 15138816, 14876672, 14614528, 14352384, 14090240, 13828096, 13565952, 13303808, 13041664, 12779520, 12517376, 12255232, 11993088, 11730944, 11468800, 11206656, 10944512, 10682368, 10420224, 10158080, 9895936, 9633792, 9371648, 9109504, 8847360, 8585216, 8323072]  # Jet(256)
          }
          frame "Rainbow_Wh" {
            w145 = u32[] [0, 262147, 589831, 851978, 1179662, 1441811, 1769495, 2031644, 2359328, 2621478, 2949163, 3276848, 3801147, 4194372, 4456520, 4522061, 4718673, 4849750, 5046363, 5177439, 5242980, 5374056, 5439597, 5505142, 5636218, 5767300, 5636232, 5701773, 5701777, 5701782, 5570714, 5505183, 5505187, 5505192, 5177521, 5111990, 5046458, 4980927, 4587720, 4456652, 4325585, 3932374, 3801306, 3604703, 3014888, 2818284, 2621681, 2359541, 2162938, 1638655, 1048831, 786687, 262399, 255, 1279, 4351, 5631, 6655, 7679, 9983, 11007, 12031, 13311, 16383, 17407, 18687, 21759, 23039, 24063, 25087, 27391, 28415, 29439, 30719, 32767, 34815, 36095, 39167, 40447, 41471, 42495, 44799, 45823, 46847, 48127, 50175, 51199, 55551, 56575, 57855, 58879, 59903, 62207, 63231, 64255, 65535, 65526, 65522, 65518, 65505, 65496, 65492, 65483, 65479, 65475, 65471, 65467, 65458, 65454, 65450, 65437, 65432, 65424, 65415, 65411, 65407, 65403, 65394, 65390, 65386, 65382, 65369, 65364, 65360, 65356, 65343, 65339, 65335, 65326, 65322, 65318, 65305, 65301, 65296, 65292, 65288, 65280, 589568, 851712, 1441536, 1703680, 1965824, 2817792, 3079936, 3407616, 3669760, 4194048, 4456192, 4783872, 5046016, 5897984, 6160128, 6422272, 7274240, 7536384, 7864064, 8126208, 8650496, 8912640, 9240320, 9502464, 10092288, 10616576, 10878720, 11730688, 11992832, 12320512, 12582656, 13106944, 13369088, 13696768, 13958912, 14548736, 14810880, 15924992, 16187136, 16449280, 16776960, 16775680, 16773632, 16772608, 16771328, 16770304, 16768256, 16766976, 16765952, 16762624, 16760576, 16759552, 16757248, 16756224, 16755200, 16753920, 16752896, 16750848, 16749568, 16748544, 16745216, 16744192, 16742144, 16739840, 16738816, 16737792, 16736512, 16734464, 16733440, 16732160, 16731136, 16727808, 16726784, 16725760, 16724736, 16721408, 16720384, 16719104, 16717056, 16716032, 16714752, 16711680, 16711680, 16711680, 16711680, 16711680, 16711680, 16711680, 16711680, 16711680, 16711680, 16711680, 16711680, 16711680, 16711680, 16711680, 16711680, 16711680, 16711680, 16777215, 16777215, 16777215, 16777215, 16777215, 16777215, 16777215, 16777215, 16777215, 16777215, 16777215, 16777215, 16777215, 16777215, 16777215, 16777215, 16777215, 16777215, 16777215, 16777215]  # Rainbow+White (237)
          }
          frame "Banded" {
            w146 = u32[] [6750846, 7013765, 7211659, 7409807, 7476371, 7411604, 7214997, 7017621, 6754453, 6490776, 6358685, 6226596, 6226092, 6226101, 6226109, 6227140, 6293961, 6296012, 6297806, 6233806, 5906635, 5512904, 4922053, 4199363, 3542212, 2950855, 2425550, 2031830, 1638622, 1376741, 1246954, 1314285, 1447407, 1975278, 2305771, 2372838, 2242272, 1783259, 1323992, 799448, 340956, 79842, 15849, 17905, 151543, 481786, 1009148, 1667324, 2193914, 2457333, 2523375, 2260968, 1801698, 1276895, 752607, 360418, 99816, 36335, 38390, 237307, 632574, 1158654, 1815550, 2275323, 2537717, 2471662, 2208487, 1683426, 1158879, 634847, 308451, 48362, 50673, 52728, 316924, 777214, 1302782, 1893373, 2352122, 2548212, 2481645, 2087398, 1628129, 1038303, 580576, 254949, 60394, 62189, 129520, 392688, 851694, 1441515, 2031078, 2423264, 2552791, 2419661, 2024898, 1499321, 974770, 516526, 190124, 60844, 62635, 129707, 458153, 982695, 1572516, 2161825, 2488475, 2552211, 2353800, 1893501, 1368177, 843623, 451166, 124759, 61010, 62797, 195401, 589383, 1113670, 1703494, 2227014, 2553410, 2551868, 2287665, 1827364, 1302294, 974603, 1040900, 1239041, 1699840, 2291200, 3013379, 3866121, 4783634, 5635611, 6355746, 6878502, 7073317, 7071521, 7004697, 6938385, 7069705, 7398403, 7858688, 8515840, 9172992, 9894916, 10550795, 11140627, 11599132, 11926051, 12055590, 11988261, 11855391, 11723032, 11788047, 11984904, 12510467, 13101824, 13759232, 14416129, 15006981, 15400460, 15728149, 15858974, 15857956, 15659558, 15395620, 15065886, 14736150, 14669582, 14800391, 15128322, 15587840, 16047616, 16441345, 16637958, 16703246, 16702743, 16570656, 16307237, 15846438, 15385379, 14924316, 14660116, 14658828, 14854661, 15182337, 15641344, 16100352, 16493826, 16690440, 16690192, 16690201, 16492833, 16163878, 15703078, 15242018, 14846235, 14647058, 14645003, 14840068, 15232513, 15690496, 16083200, 16410371, 16541193, 16541202, 16410139, 16213282, 15818789, 15292709, 14831136, 14434840, 14169616, 14166537, 14360579, 14686208, 15077888, 15404288, 15600132, 15665675, 15536665, 15342119, 15015986, 14558008, 14033211, 13507643, 13047097, 12848439, 12781367, 12911162, 13107263, 13303877, 13500748, 13501524, 13371996, 13177188, 12851050, 12393581, 11869549, 11278955, 10753384, 10293092, 9963875, 9765987, 9765220, 9764967, 9699434, 9634157, 9372526, 9111662, 8719469, 8261738]  # Banded(256)
          }
          frame "Seis" {
            w147 = u32[] [11206656, 11403264, 11599872, 11796480, 11993088, 12189696, 12386304, 12582912, 12779520, 12976128, 13172736, 13369344, 13565952, 13762560, 13959168, 14155776, 14352384, 14548992, 14745600, 14942208, 15138816, 15335424, 15532032, 15728640, 15925248, 16121856, 16318464, 16515072, 16711680, 16712448, 16713216, 16713984, 16714752, 16715520, 16716288, 16717056, 16717824, 16718592, 16719360, 16720128, 16720896, 16721664, 16722432, 16723200, 16723968, 16724736, 16725504, 16726272, 16727040, 16727808, 16728576, 16729344, 16730112, 16730880, 16731648, 16732416, 16733184, 16733952, 16734720, 16735488, 16736256, 16737024, 16737792, 16738560, 16739328, 16740096, 16740864, 16741632, 16742400, 16743168, 16743936, 16744448, 16745216, 16745984, 16746752, 16747520, 16748288, 16749056, 16749824, 16750592, 16751360, 16752128, 16752896, 16753664, 16754432, 16755200, 16755968, 16756736, 16757504, 16758272, 16759040, 16759808, 16760576, 16761344, 16762112, 16762880, 16763648, 16764416, 16765184, 16765952, 16766720, 16767488, 16768256, 16769024, 16769792, 16770560, 16771328, 16772096, 16772864, 16773632, 16774400, 16775168, 16775936, 16776704, 16776960, 16776960, 16776960, 16776960, 16776960, 16776960, 16776960, 16776960, 16776960, 16776960, 16776960, 16776960, 16776960, 16776960, 16776960, 16776960, 16776960, 16776960, 16776960, 16776960, 16776960, 16776960, 16776960, 16776960, 16776960, 16776960, 16776960, 16776960, 16645888, 16252673, 15924994, 15531779, 15138565, 14745350, 14352135, 14024456, 13631241, 13238026, 12844811, 12451596, 12123917, 11730702, 11337487, 10944272, 10551057, 10223378, 9830163, 9436948, 9043733, 8650518, 8322840, 7929625, 7536410, 7143195, 6749980, 6422301, 6029086, 5766944, 5570083, 5373222, 5176617, 4979756, 4717615, 4520753, 4324148, 4127287, 3930682, 3733821, 3471679, 3274818, 3078213, 2881352, 2684747, 2487886, 2225744, 2028883, 1832278, 1635417, 1438556, 1241950, 979553, 782948, 586087, 389482, 192620, 60784, 59509, 57979, 56704, 55173, 53642, 52367, 50836, 49305, 48030, 46499, 44968, 43694, 42163, 40888, 39357, 37826, 36551, 35020, 33489, 32214, 30684, 29409, 27878, 26347, 25072, 23541, 22010, 20735, 19965, 19195, 18426, 17912, 17142, 16372, 15603, 14833, 14319, 13549, 12780, 12010, 11240, 10726, 9957, 9187, 8417, 7647, 7134, 6364, 5594, 4824, 4055, 3541, 2771, 2001, 1232, 462]  # Seis(256)
          }
          frame "InvertSeis" {
            w148 = u32[] [462, 1232, 2001, 2771, 3541, 4055, 4824, 5594, 6364, 7134, 7647, 8417, 9187, 9957, 10726, 11240, 12010, 12780, 13549, 14319, 14833, 15603, 16372, 17142, 17912, 18426, 19195, 19965, 20735, 22010, 23541, 25072, 26347, 27878, 29409, 30684, 32214, 33489, 35020, 36551, 37826, 39357, 40888, 42163, 43694, 44968, 46499, 48030, 49305, 50836, 52367, 53642, 55173, 56704, 57979, 59509, 60784, 192620, 389482, 586087, 782948, 979553, 1241950, 1438556, 1635417, 1832278, 2028883, 2225744, 2487886, 2684747, 2881352, 3078213, 3274818, 3471679, 3733821, 3930682, 4127287, 4324148, 4520753, 4717615, 4979756, 5176617, 5373222, 5570083, 5766944, 6029086, 6422301, 6749980, 7143195, 7536410, 7929625, 8322840, 8650518, 9043733, 9436948, 9830163, 10223378, 10551057, 10944272, 11337487, 11730702, 12123917, 12451596, 12844811, 13238026, 13631241, 14024456, 14352135, 14745350, 15138565, 15531779, 15924994, 16252673, 16645888, 16776960, 16776960, 16776960, 16776960, 16776960, 16776960, 16776960, 16776960, 16776960, 16776960, 16776960, 16776960, 16776960, 16776960, 16776960, 16776960, 16776960, 16776960, 16776960, 16776960, 16776960, 16776960, 16776960, 16776960, 16776960, 16776960, 16776960, 16776960, 16776704, 16775936, 16775168, 16774400, 16773632, 16772864, 16772096, 16771328, 16770560, 16769792, 16769024, 16768256, 16767488, 16766720, 16765952, 16765184, 16764416, 16763648, 16762880, 16762112, 16761344, 16760576, 16759808, 16759040, 16758272, 16757504, 16756736, 16755968, 16755200, 16754432, 16753664, 16752896, 16752128, 16751360, 16750592, 16749824, 16749056, 16748288, 16747520, 16746752, 16745984, 16745216, 16744448, 16743936, 16743168, 16742400, 16741632, 16740864, 16740096, 16739328, 16738560, 16737792, 16737024, 16736256, 16735488, 16734720, 16733952, 16733184, 16732416, 16731648, 16730880, 16730112, 16729344, 16728576, 16727808, 16727040, 16726272, 16725504, 16724736, 16723968, 16723200, 16722432, 16721664, 16720896, 16720128, 16719360, 16718592, 16717824, 16717056, 16716288, 16715520, 16714752, 16713984, 16713216, 16712448, 16711680, 16515072, 16318464, 16121856, 15925248, 15728640, 15532032, 15335424, 15138816, 14942208, 14745600, 14548992, 14352384, 14155776, 13959168, 13762560, 13565952, 13369344, 13172736, 12976128, 12779520, 12582912, 12386304, 12189696, 11993088, 11796480, 11599872, 11403264, 11206656]  # InvertSeis(256)
          }
          frame "Jaisnd" {
            w149 = u32[] [3014783, 2949253, 2818187, 2621584, 2424982, 2228379, 2031776, 1769637, 1507497, 1245358, 917682, 655542, 327866, 190, 1218, 2757, 4041, 5580, 6863, 8402, 9941, 11480, 12763, 14301, 15840, 17378, 18916, 20198, 21736, 23274, 24556, 25837, 27375, 28656, 29938, 31219, 32500, 33781, 35062, 36343, 37368, 38649, 39673, 40698, 41723, 42747, 43772, 44796, 45821, 46589, 47613, 48381, 49406, 50174, 50942, 51710, 52478, 53502, 54270, 55038, 55806, 122110, 122878, 188926, 189695, 255999, 322303, 388607, 454911, 521215, 587519, 653823, 720127, 851966, 917499, 1048568, 1114101, 1245170, 1376239, 1441772, 1572841, 1703910, 1900515, 2031584, 2162653, 2293722, 2490327, 2621396, 2818001, 3014606, 3145676, 3342281, 3538886, 3735492, 3932097, 4194239, 4390845, 4587451, 4849593, 5046199, 5308341, 5570484, 5832626, 6029233, 6356912, 6619055, 6881199, 7143343, 7471022, 7733166, 8060847, 8388527, 8716208, 9043890, 9371571, 9764789, 10158007, 10485690, 10878908, 11337664, 11730884, 12189640, 12648397, 13172690, 13762520, 14352351, 15073256, 15990772, 16515059, 16318437, 16121818, 15990737, 15925192, 15859648, 15794105, 15794098, 15728556, 15728549, 15728543, 15794074, 15794068, 15859598, 15925129, 15925124, 15990655, 16056186, 16121717, 16252785, 16318316, 16383848, 16514916, 16580448, 16711515, 16776792, 16776276, 16775760, 16775244, 16774985, 16774469, 16773954, 16773439, 16772923, 16772408, 16771893, 16771378, 16770863, 16770093, 16769578, 16769063, 16768549, 16767778, 16767264, 16766750, 16765980, 16765465, 16764695, 16763925, 16763412, 16762642, 16761872, 16761103, 16760333, 16759564, 16758538, 16757769, 16757000, 16755975, 16755206, 16754181, 16753156, 16752131, 16751106, 16684546, 16683521, 16682497, 16681472, 16680192, 16679168, 16677888, 16676608, 16675328, 16674048, 16672768, 16671488, 16604672, 16603136, 16601856, 16600320, 16533248, 16531712, 16464640, 16463104, 16396032, 16328960, 16327168, 16260096, 16192768, 16125696, 16058368, 15991296, 15925252, 15859722, 15728657, 15663128, 15532062, 15466533, 15335467, 15204401, 15073335, 14942269, 14811203, 14680137, 14483535, 14352468, 14155865, 13959262, 13762659, 13566056, 13369452, 13172848, 12910708, 12714103, 12451962, 12189821, 11927679, 11665537, 11403394, 11075716, 10813572, 10485893, 10158212, 9830532, 9437315, 9109633, 8716415, 8323197]  # Jaisnd(256)
          }
          frame "TBD1" {
          }
        }
        n74 = property on="ImagePreview" class="IntGraph (strict)"("Color Table"=w139) -> ()  [unwired: 2 in, 2 out]
      }
      event "Start": Value Change {
        # "must check file exisance"
        n75 = event-data() -> ()  [unwired: 1 in, 1 out]
        n76 = while {
          tunnel: [w176] -> w152
          tunnel: [w172] -> w151
          stop <- w177 stop-if-true
          n77 = Not A Number/Path/Refnum?(number/path/refnum="BioMAP file path") -> (NaN/Path/Refnum?=w174:bool)
          n78 = feedback #1(path "" ("selected path")) -> (w181:path)
          n79 = case shown="True" w174 {
            tunnel: w181 -> [_ w191]
            tunnel: [w183 w190] -> w179
            tunnel: [w182 w189] -> w178
            tunnel: "BioMAP file path" -> [w183 _]
            tunnel: [w182 w184] -> w170
            frame False {
              w182 = FALSE ("cancelled")
            }
            frame True {
              n80 = Strip Path(path=w191) -> (stripped path=w186:path, name=w187:string)
              n81 = call "File Dialog2"("start path"=w186, "default name"=w187, "pattern (all files)"="*.img", "pattern label"="BioMAP Analyze v7.5") -> ("selected path"=w190:path, "exists"=w184:bool, "cancelled"=w189:bool)  [unwired: 8 in, 1 out]
            }
          }
          n82 = Compound Arithmetic op=OR(w170, w178) -> (w171:bool)
          n83 = case shown="False" w171 {
            tunnel: w179 -> [w193 _]
            tunnel: [w193 w200] -> w180
            tunnel: w181 -> [_ w200]
            tunnel: [TRUE w194] -> w177
            tunnel: [w193 path "" ("selected path")] -> w176
            tunnel: [_ w194] -> w172
            frame False {
              "Export File Path" <- w193
            }
            frame True {
              n84 = Two Button Dialog(message="No file saving?", 1:"Cancel" ("F button name (\"Cancel\")"), 2:"Set filename" ("T button name (\"OK\")")) -> (T button?=w195:bool)
              n85 = Not(x=w195) -> (.not. x?=w194:bool)
            }
          }
          n86 = feedback-in #1(w180) -> ()
        }
        n87 = property on="Start" class="Bool"("Visible"=FALSE) -> ()  [unwired: 2 in, 2 out]
        n88 = Bundle By Name(cluster=T13 {"State"=enum."SetPeakOI", "Para."=variant} ("element"), "Para."=w156) -> (w157:T13)
        n89 = Enqueue Element At Opposite End(queue=w159, element=w157) -> (queue out=w153:refnum<queue>)  [unwired: 2 in, 2 out]
        n90 = case shown="False" w151 {
          tunnel: [w168 w169] -> w154
          tunnel: w153 -> [w167 w169]
          tunnel: w152 -> [w164 _]
          frame False {
            n91 = control-ref of="MaxiMass"() -> (w160:refnum<vi>)
            n92 = control-ref of="Binning"() -> (w163:refnum<vi>)
            n93 = Bundle By Name(cluster=T13 {"State"=enum."Open", "Para."=variant} ("element"), "Para."=w164) -> (w165:T13)
            n94 = Enqueue Element At Opposite End(queue=w167, element=w165) -> (queue out=w168:refnum<queue>)  [unwired: 2 in, 2 out]
            n95 = property class="DigNum (strict)"(reference=w160, "Visible"=FALSE) -> ()  [unwired: 1 in, 2 out]
            n96 = property class="Bool (strict)"(reference=w163, "Visible"=FALSE) -> ()  [unwired: 1 in, 2 out]
          }
          frame True {
          }
        }
      }
    }
  }
  n97 = while {
    shift-right: [w218] -> _
    shift-left: w54 -> [w224]
    shift-right: [w217] -> _
    shift-left: _ -> [w223]
    tunnel: w47 -> [w222]
    tunnel: "Dynamic Params queue" -> [w214]
    shift-right: [w215] -> _
    shift-left: _ -> [w213]
    shift-right: [w212] -> _
    shift-left: _ -> [w211]
    tunnel: "Quit_UserEvent" -> [w210]
    shift-right: [w208] -> w35
    shift-left: w39 -> [w209]
    shift-right: [w204] -> _
    shift-left: _ -> [w207]
    shift-right: [w205] -> _
    shift-left: T8 {"File Header"={"Start Position"=[], "StepWidth"=[], "Dimension"=[], "SpecLength"=0}, "mzCali."=[], "m/z_Array"=[], "SampleRate"=500000000.0, "TrigDelay"=0.0, "file refnum"=refnum, "file path"=path "", "PeakOI"=[], "Binning"={"Enable"=FALSE, "BinType"=enum."ByTime", "BinWidth"=0.0, "Maximum"=0.0, "Minimum"=0.0}} ("output cluster") -> [w206]
    border: w38 -> [_]
    border: T1."Normal" ("Flag") -> [_]
    tunnel: w4 -> [w201]
    border: w2 -> [_]
    i -> [w202]
    stop <- w216 stop-if-true
    n98 = Dequeue Element(queue=w222) -> (queue out=w219:refnum<queue>, element=w220:T13, error out=w221:errorcluster)  [unwired: 2 in, 1 out]
    n99 = Unbundle By Name(w220) -> ("State"=w203:T3)
    "State" <- w203
    n100 = case shown="No Error" w221 {
      tunnel: w224 -> [w246 w1124]
      tunnel: [w245 w1124] -> w218
      tunnel: w223 -> [w244 w1123]
      tunnel: [w243 w1123] -> w217
      tunnel: w203 -> [w242 _]
      tunnel: w220 -> [w241 _]
      tunnel: w219 -> [w240 _]
      tunnel: [w239 TRUE] -> w216
      tunnel: [w238 w1121] -> w215
      tunnel: w214 -> [w237 _]
      tunnel: w213 -> [w236 w1121]
      tunnel: [w235 w1120] -> w212
      tunnel: w211 -> [w234 w1120]
      tunnel: w210 -> [w233 _]
      tunnel: w209 -> [w232 w1119]
      tunnel: [w226 w1119] -> w208
      tunnel: w207 -> [w231 w1117]
      tunnel: w206 -> [w230 w1118]
      tunnel: [w229 w1118] -> w205
      tunnel: [w228 w1117] -> w204
      tunnel: w201 -> [w225 _]
      frame No Error {
        n101 = case "Proc. Core" shown="\"CheckEndCondition\"" w242 {
          selector: w242 -> [_ w332 w389 _ w639 w656 _ _ _ _ _ _ _]
          tunnel: w246 -> [w274 w294 w403 w451 w629 w661 w669 w837 w854 w901 w922 w1106 w1116]
          tunnel: [w263 w336 w385 w450 w629 w661 w669 w837 w854 w901 w922 w1106 w1116] -> w245
          tunnel: [w279 0 w383 w448 w613 w653 w662 w838 w869 w900 w968 w1097 w1115] -> w243
          tunnel: w244 -> [w279 _ w383 w448 w620 w653 w662 w838 w869 w900 w968 w1097 w1115]
          tunnel: w241 -> [_ w315 w391 w472 w640 w657 _ _ _ w892 w961 w1105 _]
          tunnel: w240 -> [_ w333 w392 w473 w641 w658 w671 _ _ _ _ _ _]
          tunnel: [_ _ _ _ _ _ _ _ TRUE _ _ _ _] -> w239
          tunnel: [w278 w330 w387 w471 w636 w655 w682 w835 w867 w895 w964 w1098 w1114] -> w238
          tunnel: w237 -> [_ _ w394 _ _ _ _ _ w860 _ _ _ _]
          tunnel: w236 -> [w278 _ w387 w471 w637 w655 w682 w835 w867 w895 w964 w1098 w1114]
          tunnel: [w277 w301 w384 w447 w638 w654 w681 w833 w866 w899 w967 w1096 w1113] -> w235
          tunnel: w234 -> [w277 _ w384 w447 w638 w654 w681 w833 w866 w899 w967 w1096 w1113]
          tunnel: w233 -> [_ _ _ _ _ _ _ _ w865 _ _ _ _]
          tunnel: w232 -> [w276 _ w382 w470 _ w652 w680 w827 w856 w898 w966 w1107 w1112]
          tunnel: [w276 w325 w381 w470 w635 w652 w680 w827 w857 w898 w966 w1107 w1112] -> w227
          tunnel: w231 -> [_ w292 w379 w468 w619 w650 w679 w828 w858 w896 w965 w1109 w1110]
          tunnel: w230 -> [w275 w295 w380 w457 w616 w651 w668 w829 w859 w897 w921 w1103 w1111]
          tunnel: [w254 w326 w380 w457 w616 w651 w668 w829 w859 w897 w921 w1108 w1111] -> w229
          tunnel: [w255 w292 w379 w469 w618 w650 w679 w828 w858 w896 w965 w1109 w1110] -> w228
          tunnel: w225 -> [_ _ _ _ _ _ _ _ w855 _ _ _ _]
          frame "Initialize" {
            w261 = sgl -1.0  # NaN cannot be "-1"  when write to disk
            w262 = 0  # Scan#, should not be reset to 0 in "open", for 3D imaging.
            # "floating number to integar number conversion error correction, \nlegacy part, which is not need in multiple line construction"
            n102 = Unbundle By Name(w274) -> ("InfoBarRef."=w247:refnum<vi>, "File Header.SpecLength"=w270:i32, "File Header"=w269:T9, "mzCali."=w273:dbl[], "SampleRate"=w271:T10, "TrigDelay"=w272:dbl)
            n103 = in-place "Compensate error in float-point number calculation" {
              n104 = in-place-cluster #2(w269) -> ("StepWidth"=w282:dbl[], "Start Position"=w284:dbl[])
              n105 = Multiply(x=w282, y=0.001) -> (x*y=w281:dbl[])
              n106 = in-place {
                in-place-border: w281 -> [w286]
                n107 = in-place-split #3(w284, 2) -> (w289:dbl[], w287:dbl[])
                n108 = Subtract(x=w289, y=w286) -> (x-y=w288:dbl[])
                n109 = in-place-split #3(w288, w287) -> (w283:dbl[])  [unwired: 1 out]
              }
              n110 = in-place-cluster #2("StepWidth"=w282, "Start Position"=w283) -> (w268:T9)
            }
            n111 = property class="Str"(reference=w247, "Value"="Image preview starts after the 8th line scans.") -> ()  [unwired: 1 in, 2 out]
            n112 = call "CalcMzArray.vi"("TrigDelay"=w272, "Sample Rate"=w271, "Depth"=w270, "mzCali. (a/b/c)"=w273) -> ("mzArray"=w264:dbl[])  [unwired: 7 in]
            n113 = Bundle By Name(cluster=w274, "Scan#"=w262) -> (w263:T14)
            n114 = Bundle By Name(cluster=w275, "Binning.BinType"=BinType."ByMass", "Binning.BinWidth"=0.1, "Binning.Minimum"=0.0, "File Header.SpecLength"=w270, "m/z_Array"=w264, "File Header"=w268, "mzCali."=w273, "SampleRate"=w271, "TrigDelay"=w272) -> (w254:T8)
            n115 = Unbundle By Name(w254) -> ("File Header.SpecLength"=w252:i32, "File Header.Dimension"=w253:i32[])
            n116 = Index Array(array=w253) -> (element #1=w251:i32, element #2=w250:i32)  [unwired: 2 in]
            n117 = Compound Arithmetic op=MULTIPLY(w252, w251, 8 ("dimension size")) -> (w260:i32)
            n118 = Compound Arithmetic op=MULTIPLY(w250, 8 ("dimension size")) -> (w257:i32)
            n119 = To Single Precision Float(number=w261) -> (single precision float=w249:sgl)
            n120 = Initialize Array(w249, w260) -> (w255:sgl[])
            n121 = Initialize Array(0, w257) -> ()  [unwired: 1 out]
          }
          frame "Open" {
            w297 = "ActionCallBack" ("name (unnamed)")
            # "check:\n\nsecdata interpolation on?\nMultiple record ?"
            # "8192x32KB*4 = 1GB\n!! attention:\nshould be big"
            # "Can -1 be made NaN??"
            # "Save Header + MzArray first.\nIn case of program crash, \nBioMAP v3.8+ will load partial file just fine."
            n122 = Increment(x=w332) -> (x+1=w334:T3)
            n123 = Bundle By Name(cluster=w315, "State"=w334) -> (w335:T13)
            n124 = Unbundle By Name(w315) -> ("Para."=w314:variant)
            n125 = Enqueue Element(queue=w333, element=w335) -> ()  [unwired: 2 in, 3 out]
            n126 = Variant To Data(type=path "" ("selected path"), Variant=w314) -> (data=w306:path, error out=w310:errorcluster)  [unwired: 1 in]
            n127 = Unbundle By Name(w294) -> ("MultiRec Mode"=w293:bool)
            n128 = Open/Create/Replace File(file path (use dialog)=w306, error in=w310, operation (0:open)=T18."create", access (0:read/write)=enum16{"read/write", "read-only", "write-only"}."write-only") -> (refnum out=w304:refnum<file>, error out=w308:errorcluster)  [unwired: 2 in, 1 out]
            n129 = Obtain Queue(max queue size (-1, unlimited)=8192, name (unnamed)="Imaging_Buffer", element data type=T17 {"tickcount"=0, "Signal"=[], "SecondaryData"=[], "Flag"=enum."Normal", "Segment#"=0} ("Signal_Typedef")) -> (queue out=w301:refnum<queue>)  [unwired: 2 in, 2 out]
            n130 = Obtain Queue(name (unnamed)=w297, element data type=w297) -> (queue out=w296:refnum<queue>)  [unwired: 3 in, 2 out]
            n131 = case shown="Error" w308 {
              selector: w308 -> [_ w370]
              tunnel: [_ w364] -> w307
              tunnel: w306 -> [w363 w366]
              tunnel: [w363 w366] -> w305
              tunnel: w304 -> [w362 w365]
              tunnel: [w362 w365] -> w303
              frame No Error {
              }
              frame Error {
                n132 = Two Button Dialog(message="Error when create image file.", 1:"No saving" ("F button name (\"Cancel\")"), 2:"Ignore" ("T button name (\"OK\")")) -> ()  [unwired: 1 out]
                n133 = call <vilib>:"Clear Errors.vi"("error in (no error)"=w370) -> ("error out"=w364:errorcluster)  [unwired: 5 in, 1 out]
              }
            }
            n134 = case shown="True" w293 {
              tunnel: w301 -> [w349 w351]
              tunnel: w294 -> [w348 w353]
              tunnel: w296 -> [w337 w352]
              frame False {
                n135 = Unbundle By Name(w348) -> ("ControlRefs.ProcCore_CtrlQueue"=w344:refnum<queue>)
                n136 = Bundle("queue out"=w349, "queue out"=w337) -> (w340:T26)  [unwired: 1 in]
                n137 = Bundle By Name(cluster=T19 {"Command"=enum."SetWriterRef", "Params"=variant} ("element"), "Command"=ProcessStates."SetWriterRef", "Params"=w340) -> (w346:T19)
                n138 = Enqueue Element "Set Data queue"(queue=w344, element=w346) -> (queue out=w342:refnum<queue>, error out=w339:errorcluster)  [unwired: 2 in, 1 out]
                n139 = Dequeue Element(queue=w337, error in (no error)=w339) -> (error out=w338:errorcluster)  [unwired: 1 in, 3 out]
                n140 = Enqueue Element "Start Send Data"(queue=w342, element=T19 {"Command"=enum."StartSave", "Params"=variant}, error in (no error)=w338) -> (error out=w341:errorcluster)  [unwired: 1 in, 2 out]
                n141 = call <vilib>:"Clear Errors.vi"("error in (no error)"=w341) -> ()  [unwired: 5 in, 2 out]
              }
              frame True {
                n142 = Bundle("queue out"=w351, "queue out"=w352) -> ()  [unwired: 1 in, 1 out]
                n143 = Unbundle By Name(w353) -> ("ControlRefs.MainDAQCoreQueue"=w357:refnum<queue>)
                n144 = Bundle By Name(cluster=T21 {"GenericDAQ State"=enum."SetDynamicBuffer_", "Variant"=variant} ("element"), "Variant"=w351) -> (w354:T21)
                n145 = Enqueue Element "Set Data queue"(queue=w357, element=w354) -> (error out=w356:errorcluster)  [unwired: 2 in, 2 out]
                n146 = disable-structure shown="Enabled" {
                  disable-tunnel: w356 -> [w360 w361]
                  disable-tunnel: w352 -> [w359 _]
                  disable-tunnel: [w358 w361] -> w350
                  frame Disabled {
                    n147 = Dequeue Element(queue=w359, error in (no error)=w360) -> (error out=w358:errorcluster)  [unwired: 1 in, 3 out]
                  }
                  frame Enabled {
                  }
                }
                n148 = Flush Queue(queue=w351, error in (no error)=w350) -> ()  [unwired: 3 out]
              }
            }
            n149 = Unbundle By Name(w295) -> ("File Header.Dimension"=w328:i32[])
            n150 = Index Array(array=w328) -> (element #1=w291:i32, element #2=w327:i32)  [unwired: 2 in]
            n151 = Unbundle By Name(w295) -> ("Binning.BinWidth"=w320:dbl, "Binning.Minimum"=w321:dbl, "m/z_Array"=w322:dbl[], "Binning.BinType"=w323:T11)
            n152 = Initialize Array "Potential Insufficient Memory Source"(sgl nan, w291, w327, 32 ("dimension size")) -> (w330:sgl[][][])
            n153 = Bundle By Name(cluster=w295, "Binning.Maximum"="MaxiMass", "Binning.Enable"="Binning", "file path"=w305, "file refnum"=w303) -> (w326:T8)
            n154 = call "SpectrumBinning_NoGraph.vi"("XScale.Maximum"="MaxiMass", "BinType"=w323, "BinWidth"=w320, "Enable"="Binning", "Signal"=w322, "m/z Array"=w322, "XScale.Minimum"=w321) -> ("m/z Array"=w319:dbl[])  [unwired: 2 in, 2 out]
            n155 = Array Size(array=w319) -> (size(s)=w318:i32)
            n156 = Bundle By Name(cluster=w326, "File Header.SpecLength"=w318, "m/z_Array"=w319) -> (w324:T8)
            n157 = Unbundle By Name(w307) -> ("status"=w309:bool)
            n158 = Not(x=w309) -> (.not. x?=w302:bool)
            n159 = call "WriteHeader+MzArray(AnalyzeV75).vi"("error in (no error)"=w307, "ImageConvParams"=w324) -> ("error out"=w325:errorcluster)  [unwired: 9 in]
            n160 = Bundle By Name(cluster=w294, "Save?"=w302) -> (w336:T14)
          }
          frame "PrepScanParams" {
            n161 = Increment(x=w389) -> (x+1=w388:T3)
            n162 = Bundle By Name(cluster=w391, "State"=w388) -> (w390:T13)
            n163 = Unbundle By Name(w403) -> ("Scan#"=w395:i32, "ControlRefs"=w376:T5, "File Header.Dimension"=w375:i32[])
            n164 = Enqueue Element(queue=w392, element=w390) -> ()  [unwired: 2 in, 3 out]
            n165 = Index Array(array=w375) -> (element=w374:i32)  [unwired: 1 in]
            n166 = Increment(x=w395) -> (x+1=w402:i32)
            n167 = Bundle By Name(cluster=w403, "Scan#"=w402) -> (w385:T14)
            n168 = Compound Arithmetic op=MULTIPLY(w374, 5 ("value"), 1 ("value")) -> (w371:i32)
            "segment #" <- w371
            n169 = Equal To 0?(x=w395) -> (x = 0?=w404:bool)
            n170 = case shown="False" w404 {
              tunnel: w403 -> [w416 w442]
              tunnel: [w406 w438] -> w400
              tunnel: [w410 w441] -> w399
              tunnel: [w409 w440] -> w398
              tunnel: [w408 w439] -> w397
              tunnel: w395 -> [_ w423]
              tunnel: w383 -> [_ _]
              frame True {
                w405 = 0
                # "Initial scan, stick to orignal parameter"
                n171 = Unbundle By Name(w416) -> ("HighSpeed"=w409:dbl, "ScanSpeed"=w408:dbl, "File Header"=w411:T9)
                n172 = Unbundle By Name(w411) -> ("Start Position"=w406:dbl[], "StepWidth"=w414:dbl[], "Dimension"=w415:i32[])
                n173 = Index Array(array=w414, index=w405) -> (element=w413:dbl)
                n174 = Index Array(array=w415, index=w405) -> (element=w412:i32)
                n175 = Multiply(x=w413, y=w412) -> (x*y=w407:dbl)
                n176 = in-place {
                  in-place-border: w407 -> [w418]
                  n177 = in-place-array #4(w406, w405) -> (w419:dbl)
                  n178 = Add(x=w419, y=w418) -> (x+y=w417:dbl)
                  n179 = in-place-array #4(w417) -> (w410:dbl[])  [unwired: 1 out]
                }
              }
              frame False {
                w420 = 1
                w429 = 0 ("index")
                n180 = Unbundle By Name(w442) -> ("HighSpeed"=w440:dbl, "ScanSpeed"=w439:dbl, "File Header"=w431:T9)
                n181 = Unbundle By Name(w431) -> ("Start Position"=w424:dbl[], "StepWidth"=w436:dbl[], "Dimension"=w437:i32[])
                n182 = Index Array(array=w424, index #1=w429, index #2=w420) -> (element #1=w435:dbl, element #2=w426:dbl)
                n183 = Index Array(array=w436, index #1=w429, index #2=w420) -> (element #1=w433:dbl, element #2=w428:dbl)
                n184 = Index Array(array=w437, index #1=w429, index #2=w420) -> (element #1=w432:i32, element #2=w422:i32)
                n185 = Quotient & Remainder "Circle Y #"(x=w423, y=w422) -> (x-y*floor(x/y)=w421:i32)  [unwired: 1 out]
                n186 = Multiply(x=w433, y=w432) -> (x*y=w434:dbl)
                n187 = Multiply(x=w428, y=w421) -> (x*y=w427:dbl)
                n188 = Add "X"(x=w435, y=w434) -> (x+y=w430:dbl)
                n189 = Add "Y"(x=w426, y=w427) -> (x+y=w425:dbl)
                n190 = in-place {
                  in-place-border: w430 -> [w444]
                  in-place-border: w425 -> [w443]
                  # "X"
                  # "Y"
                  n191 = in-place-array #5(w424, w420) -> ()  [unwired: 1 out]
                  n192 = in-place-array #6(w424, w429, w420) -> ()  [unwired: 2 out]
                  n193 = in-place-array #5(w443) -> (w438:dbl[])  [unwired: 1 out]
                  n194 = in-place-array #6(w444, w443) -> (w441:dbl[])  [unwired: 2 out]
                }
              }
            }
            n195 = Bundle By Name(cluster=cluster{"Queue cluster":T5, "Segment#":i32} {"Queue cluster"={"LaserCtrlMethod"=enum."SRS_DG535", "Apps"=refnum, "MainDAQCoreQueue"=refnum, "Micos"=refnum, "ESP300"=refnum, "SMC100"=refnum, "SRS DG535"=refnum, "BNC"=refnum, "SDG_ii"=refnum, "NI-USB_DAQmx"=refnum, "ProcCore_CtrlQueue"=refnum, "WriterCtrl"=refnum, "WriterSIG"=refnum, "Feedback"=refnum, "EPM2000"=refnum, "InfoRef"=refnum, "AppsLock"=refnum, "ProcCore_SignalBuffer"=refnum}, "Segment#"=0}, "Queue cluster"=w376, "Segment#"=w371) -> (w377:cluster{"Queue cluster":T5, "Segment#":i32})
            n196 = Bundle By Name(cluster=T23 {"Line Start"=[], "Line End"=[], "HighSpeed"=0.0, "ScanSpeed"=0.0, "KeepStill(ms)"=0, "SecendaryParams"=variant}, "HighSpeed"=w398, "ScanSpeed"=w397, "Line Start"=w400, "Line End"=w399, "KeepStill(ms)"=u32 0 ("Wait(ms)"), "SecendaryParams"=w377) -> (w393:T23)
            n197 = Enqueue Element "Send scan params"(queue=w394, element=w393) -> (error out=w386:errorcluster)  [unwired: 2 in, 2 out]
            n198 = Merge Errors(w386, w382) -> (w381:errorcluster)
            n199 = call <vilib>:"Clear Errors.vi"("error in (no error)"=w386) -> ()  [unwired: 5 in, 2 out]
          }
          frame "WaitData" {
            w463 = u32 139  # A prime number to minimize artifact
            # "Line#, goes with Flush counts"
            # "Potential dead lock"
            # "Need EOF detection, \nAnd set Y Dimension to current value"
            n200 = Dequeue Element "WaitSpectra"(queue=w447) -> (element=w446:T17)  [unwired: 2 in, 3 out]
            n201 = Unbundle By Name(w446) -> ("tickcount"=w458:u32, "SecondaryData"=w455:dbl[], "Signal"=w459:sgl[], "Segment#"=w445:i32, "Flag"=w456:T1)
            "Flag" <- w456
            n202 = Unbundle By Name(w457) -> ("File Header.Dimension"=w453:i32[], "File Header.SpecLength"=w454:i32, "File Header.Start Position"=w461:dbl[], "File Header.StepWidth"=w462:dbl[])
            n203 = To Single Precision Float(number=w445) -> (single precision float=w452:sgl)
            n204 = feedback-in #7(w456) -> ()
            n205 = feedback #7() -> (w460:T1)
            n206 = Multiply(x=w459, y=w452) -> (x*y=w449:sgl[])
            n207 = case "Average Spectra in a single pixel" shown="\"Normal\"" w456 {
              tunnel: w473 -> [w481 w519 _ w537]
              tunnel: w472 -> [_ w518 _ w536]
              tunnel: w468 -> [w495 w515 w525 w543]
              tunnel: [w495 w515 w525 w542] -> w469
              tunnel: w449 -> [_ _ _ w539]
              tunnel: w455 -> [_ _ _ w555]
              tunnel: w462 -> [_ _ _ w554]
              tunnel: w461 -> [_ _ _ w553]
              tunnel: w460 -> [_ _ _ _]
              tunnel: w458 -> [_ _ _ _]
              tunnel: w454 -> [_ _ _ w540]
              tunnel: w453 -> [w491 w510 _ w545]
              tunnel: w452 -> [_ _ _ w538]
              tunnel: w451 -> [w493 w512 w524 w534]
              tunnel: [w494 w513 w524 w534] -> w450
              tunnel: w448 -> [w488 _ _ _]
              tunnel: w447 -> [_ _ _ w530]
              tunnel: w446 -> [_ _ _ w529]
              tunnel: w445 -> [_ _ _ _]
              frame "LineEnd" {
                # "End of Line"
                n208 = Index Array(array=w491) -> (element #2=w489:i32)  [unwired: 2 in, 1 out]
                n209 = Unbundle By Name(w493) -> ("EOL_cts"=w492:i32)
                n210 = Increment(x=w492) -> (x+1=w486:i32)
                "#EOL" <- w486
                n211 = Quotient & Remainder(x=w486, y=w489) -> (x-y*floor(x/y)=w490:i32)  [unwired: 1 out]
                n212 = Bundle By Name(cluster=w493, "EOL_cts"=w486) -> (w494:T14)
                n213 = Equal To 0?(x=w490) -> (x = 0?=w482:bool)
                n214 = case shown="False" w482 {
                  tunnel: w481 -> [w501 w502]
                  tunnel: [w500 w502] -> w480
                  frame False {
                    n215 = Enqueue Element(queue=w501, element=T13 {"State"=enum."PrepScanParams", "Para."=variant}) -> (queue out=w500:refnum<queue>)  [unwired: 2 in, 2 out]
                  }
                  frame True {
                  }
                }
                n216 = Subtract(x=w489, y=w488) -> (x-y=w487:i32)
                n217 = case shown="True" w482 {
                  tunnel: w480 -> [_ w504]
                  tunnel: w487 -> [_ w503]
                  frame False {
                  }
                  frame True {
                    n218 = for {
                      N: w503 -> [_]
                      tunnel: w504 -> [w505]
                      n219 = Enqueue Element(queue=w505, element=T13 {"State"=enum."Flush", "Para."=variant}) -> ()  [unwired: 2 in, 3 out]
                    }
                  }
                }
                n220 = call <vilib>:"High Resolution Relative Seconds.vi"() -> ("relative seconds"=w483:dbl)
                n221 = call <vilib>:"High Resolution Relative Seconds.vi"() -> ("relative seconds"=w498:dbl)
                "EOL time" <- w498
                n222 = local read "line start time"() -> (w497:dbl)
                n223 = feedback #8() -> (w484:dbl)  [unwired: 1 in]
                n224 = Subtract(x=w483, y=w484) -> (x-y=→"EOL interval":dbl)
                n225 = feedback-in #8(w483) -> ()
                n226 = Subtract(x=w498, y=w497) -> (x-y=→"line time":dbl)
              }
              frame "LineStart" {
                # "New Line"
                n227 = Unbundle By Name(w512) -> ("SOL_cts"=w514:i32)
                n228 = Index Array(array=w510) -> (element #2=w508:i32)  [unwired: 2 in, 1 out]
                n229 = Increment(x=w514) -> (x+1=w509:i32)
                "#SOL" <- w509
                n230 = Bundle By Name(cluster=w512, "SOL_cts"=w509) -> (w513:T14)
                n231 = Quotient & Remainder(x=w509, y=w508) -> (x-y*floor(x/y)=w511:i32)  [unwired: 1 out]
                n232 = Equal To 0?(x=w511) -> ()  [unwired: 1 out]
                n233 = call <vilib>:"High Resolution Relative Seconds.vi"() -> ("relative seconds"=→"line start time":dbl)
                n234 = case shown="True" TRUE {
                  tunnel: w519 -> [w522 w523]
                  tunnel: [w521 w523] -> w516
                  frame False {
                    n235 = Enqueue Element(queue=w522, element=T13 {"State"=enum."PrepScanParams", "Para."=variant}) -> (queue out=w521:refnum<queue>)  [unwired: 2 in, 2 out]
                  }
                  frame True {
                  }
                }
                n236 = Enqueue Element "Implied \"WaitData\""(queue=w516, element=w518) -> ()  [unwired: 2 in, 3 out]
              }
              frame Default {
                n237 = One Button Dialog(message="Defaults in Signal averager in Imaging_proc,\nwhy a non \"Normal, linestart, or lineend\" detected") -> ()  [unwired: 1 in, 1 out]
              }
              frame "Normal" {
                # "BufferFull rec"
                # "Y/8"
                # "Normal Spectra"
                n238 = Index Array(array=w545) -> (element=w544:i32)  [unwired: 1 in]
                n239 = Index Array(array=w553) -> (element #1=w562:dbl, element #2=w563:dbl)  [unwired: 2 in]
                n240 = Index Array(array=w554) -> (element #1=w564:dbl, element #2=w565:dbl)  [unwired: 2 in]
                n241 = Index Array(array=w555) -> (element #1=w552:dbl, element #2=w566:dbl)  [unwired: 2 in]
                n242 = Subtract "Y"(x=w566, y=w563) -> (x-y=w559:dbl)
                n243 = Subtract "X"(x=w552, y=w562) -> (x-y=w560:dbl)
                n244 = Divide(x=w559, y=w565) -> (x/y=w558:dbl)
                n245 = Divide(x=w560, y=w564) -> (x/y=w561:dbl)
                n246 = Round Toward -Infinity(1:w561) -> (0:w556:dbl)
                n247 = Round Toward -Infinity(1:w558) -> (0:w557:dbl)
                n248 = To Long Integer(number=w556) -> (32bit integer=w527:i32)
                n249 = To Long Integer(number=w557) -> (32bit integer=w533:i32)
                n250 = Quotient & Remainder(x=w533, y=8) -> (x-y*floor(x/y)=w532:i32, floor(x/y)=w531:i32)
                n251 = Multiply(x=w540, y=w527) -> (x*y=w547:i32)
                n252 = Compound Arithmetic op=MULTIPLY(w540, w544, w532) -> (w546:i32)
                n253 = Add(x=w547, y=w546) -> (x+y=w541:i32)
                n254 = feedback #9() -> (w550:i32[])
                n255 = Index Array(array=w550, index=w532) -> (element=w551:i32)
                n256 = Subtract(x=w531, y=w551) -> (x-y=w528:i32)
                n257 = Subtract(x=w531, y=w551) -> (x-y=w549:i32)
                n258 = case shown="0, 1" w528 {
                  tunnel: w543 -> [w570 w571 w576]
                  tunnel: [w570 w571 w577] -> w542
                  tunnel: w541 -> [_ _ w572]
                  tunnel: w540 -> [_ _ w575]
                  tunnel: w539 -> [_ _ w584]
                  tunnel: w538 -> [_ _ w583]
                  frame -1 {
                    # "invalid data,\nout of bufffer range\nimplecation of too much vibration or \ninternal error"
                    n259 = feedback #10(0) -> (w569:i32)
                    n260 = Increment(x=w569) -> (x+1=w567:i32)
                    "discarded ct" <- w567
                    n261 = feedback-in #10(w567) -> ()
                  }
                  frame 2, Default {
                  }
                  frame 0, 1 {
                    n262 = Array Subset(array=w576, index=w572, length=w575) -> (w574:sgl[])
                    n263 = in-place {
                      in-place-border: w583 -> [w585]
                      n264 = in-place-array #11(w584, 0) -> ()  [unwired: 1 out]
                      n265 = in-place-array #11(w585) -> (w580:sgl[])  [unwired: 1 out]
                    }
                    n266 = Index Array(array=w574) -> (element=w579:sgl)  [unwired: 1 in]
                    n267 = Greater Than 0?(x=w579) -> (x > 0?=w578:bool)
                    n268 = Add(x=w574, y=w580) -> (x+y=w581:sgl[])
                    n269 = Select(t=w581, s=w578, f=w580) -> (s? t:f=w573:sgl[])
                    n270 = Replace Array Subset(array=w576, new element=w573, index=w572) -> (w577:sgl[])
                    n271 = Index Array(array=w573) -> ()  [unwired: 1 in, 1 out]
                  }
                }
                n272 = case shown="1" w549 {
                  selector: w549 -> [_ _ _ w605]
                  tunnel: w531 -> [_ w594 w603 _]
                  tunnel: w550 -> [w588 w593 w602 w606]
                  tunnel: [w588 w592 w601 w606] -> w535
                  tunnel: w532 -> [_ w591 w600 _]
                  tunnel: w537 -> [w587 w590 w599 w608]
                  tunnel: w536 -> [w586 _ _ w607]
                  tunnel: w530 -> [_ _ w597 _]
                  tunnel: w529 -> [_ _ w596 _]
                  frame 0 {
                    n273 = Enqueue Element "\"WaitData\""(queue=w587, element=w586) -> ()  [unwired: 2 in, 3 out]
                  }
                  frame 1 {
                    # "Flush"
                    n274 = in-place {
                      in-place-border: w594 -> [w595]
                      n275 = in-place-array #12(w593, w591) -> ()  [unwired: 1 out]
                      n276 = in-place-array #12(w595) -> (w592:i32[])  [unwired: 1 out]
                    }
                    n277 = Enqueue Element(queue=w590, element=T13 {"State"=enum."Flush", "Para."=variant}) -> ()  [unwired: 2 in, 3 out]
                  }
                  frame 2.. {
                    n278 = in-place {
                      in-place-border: w603 -> [w604]
                      n279 = in-place-array #13(w602, w600) -> ()  [unwired: 1 out]
                      n280 = in-place-array #13(w604) -> (w601:i32[])  [unwired: 1 out]
                    }
                    n281 = Enqueue Element(queue=w599, element=T13 {"State"=enum."Flush", "Para."=variant}) -> ()  [unwired: 2 in, 3 out]
                    n282 = Enqueue Element At Opposite End(queue=w597, element=w596) -> ()  [unwired: 2 in, 3 out]
                  }
                  frame Default {
                    n283 = Enqueue Element "\"WaitData\""(queue=w608, element=w607) -> ()  [unwired: 2 in, 3 out]
                    n284 = disable-structure shown="Enabled" {
                      frame Disabled {
                        n285 = Two Button Dialog(message="too much vibration", 1:"OK" ("F button name (\"Cancel\")"), 2:"Quit ChiMS" ("F button name (\"Cancel\")")) -> (T button?=w611:bool)
                        n286 = Stop(stop? (T)=w611) -> ()
                      }
                      frame Enabled {
                      }
                    }
                    "Numeric" <- w605
                  }
                }
                n287 = feedback-in #9(w535) -> ()
              }
            }
            n288 = Tick Count (ms)() -> (millisecond timer value=w464:u32)
            n289 = Less?(x=w463, y=w464) -> (x < y?=w465:bool)
            n290 = feedback #14() -> (w466:u32)
            n291 = case "raw MS refresh" shown="True" w465 {
              tunnel: w449 -> [_ w478]
              tunnel: w464 -> [_ w479]
              tunnel: [w474 w479] -> w467
              tunnel: w466 -> [w474 _]
              tunnel: w457 -> [_ w476]
              frame False {
              }
              frame True {
                n292 = Unbundle By Name(w476) -> ("m/z_Array"=w477:dbl[])
                n293 = Bundle("m/z_Array"=w477, w478) -> (→"MS (Raw)":cluster{"m/z_Array":dbl[], sgl[]})  [unwired: 1 in]
              }
            }
            n294 = feedback-in #14(w467) -> ()
          }
          frame "Flush" {
            n295 = Increment(x=w639) -> (x+1=w614:T3)
            n296 = Unbundle By Name(w629) -> ("InfoBarRef."=w628:refnum<vi>)
            n297 = Bundle By Name(cluster=w640, "State"=w614) -> (w615:T13)
            n298 = Enqueue Element(queue=w641, element=w615) -> (queue out=w634:refnum<queue>, error out=w633:errorcluster)  [unwired: 2 in, 1 out]
            n299 = property class="Str"(reference=w628, "Value"="Flushing: Don't Panic. ") -> (reference out=w627:refnum<vi>, error out=w617:errorcluster)  [unwired: 1 in]
            n300 = property on="PeakOI #" class="DigNum (strict)"() -> ("Value"=w630:i32)  [unwired: 2 in, 2 out]
            n301 = Bundle By Name(cluster=T13 {"State"=enum."Refresh_Image", "Para."=variant} ("element"), "Para."=w630) -> (w631:T13)
            n302 = flat-sequence {
              tunnel: w634 -> [w649]
              tunnel: w633 -> [w648]
              tunnel: w631 -> [w647]
              tunnel: [w646] -> _
              tunnel: [w645] -> w622
              frame #0 {
                n303 = Enqueue Element(queue=w649, element=w647, error in (no error)=w648) -> (error out=w646:errorcluster)  [unwired: 1 in, 2 out]
                n304 = call <vilib>:"High Resolution Relative Seconds.vi"() -> ("relative seconds"=w645:dbl)
              }
            }
            n305 = call "ImageConstructer(MultilineBuffer).vi"("Image Params"=w616, "Image in"=w637, "error in"=w617, "ImageBuffer in"=w619, "Y_img"=w620) -> ("error out"=w625:errorcluster, "ImageBuffer out"=w618:sgl[], "Image out"=w636:dbl[][][])  [unwired: 2 in, 2 out]
            n306 = flat-sequence {
              tunnel: [w644] -> w635
              tunnel: w625 -> [w643]
              tunnel: [w642] -> w623
              frame #0 {
                n307 = call <vilib>:"High Resolution Relative Seconds.vi"() -> ("relative seconds"=w642:dbl)
                n308 = call <vilib>:"General Error Handler.vi"("error in (no error)"=w643) -> ("error out"=w644:errorcluster)  [unwired: 10 in, 4 out]
              }
            }
            n309 = Subtract(x=w623, y=w622) -> (x-y=→"flushing time":dbl)
            n310 = Increment(x=w620) -> (x+1=w613:i32)
            "Line# (Y_Img)" <- w613
            n311 = property class="Str"(reference=w627, error in=w625, "Value"="") -> ()  [unwired: 2 out]
          }
          frame "ScanResult" {
            # "For comapatibility with other static subprogram, drive the loop going"
            n312 = Increment(x=w656) -> (x+1=w659:T3)
            n313 = Bundle By Name(cluster=w657, "State"=w659) -> (w660:T13)
            n314 = Enqueue Element(queue=w658, element=w660) -> ()  [unwired: 2 in, 3 out]
          }
          frame "CheckEndCondition" {
            w676 = 2  # axis:Z
            w683 = 1  # axis:Y
            # "Some bug may exist"
            # "fitted for 3D imaing, \nmay not fit for binary file conversion"
            # "Add condition:\nreader quit due to file ends"
            n315 = Unbundle By Name(w669) -> ("File Header.Dimension"=w684:i32[])  [unwired: 1 out]
            n316 = Index Array(array=w684, index #1=w683, index #2=w676) -> (element #1=w674:i32, element #2=w666:i32)
            n317 = Multiply(x=w674, y=w666) -> (x*y=w675:i32)
            n318 = Quotient & Remainder(x=w662, y=w674) -> (x-y*floor(x/y)=w667:i32, floor(x/y)=w665:i32)
            n319 = Subtract(x=w675, y=w662) -> (x-y=→"remaining lines":i32)
            n320 = Equal To 0? "2D_Image finished?"(x=w667) -> (x = 0?=w664:bool)
            n321 = Greater Or Equal? "3D_Image finished"(x=w665, y=w666) -> (x >= y?=w663:bool)
            n322 = case "One Image Finish" shown="False" w664 {
              tunnel: w665 -> [_ w687]
              tunnel: [T13 {"State"=enum."WaitData", "Para."=variant} w697] -> w672
              tunnel: w671 -> [w685 w703]
              tunnel: [w685 w702] -> w670
              tunnel: w668 -> [_ w700]
              frame False {
                # "prepscanparams is done \npreviously in waitdata:endofline"
                # "Continue next line scan"
              }
              frame True {
                # "If the file exist, error will be thrown out \nand will crash the expt !, proper error handling needed"
                # "to be done"
                # "A signal image finished in 3D imaging."
                n323 = Unbundle By Name(w700) -> ("file path"=w698:path)
                n324 = Enqueue Element(queue=w703, element=T13 {"State"=enum."Close", "Para."=variant}) -> (queue out=w702:refnum<queue>)  [unwired: 2 in, 2 out]
                n325 = Strip Path(path=w698) -> (stripped path=w699:path, name=w688:string)
                n326 = Format Value(string ("")="_", format string="%04d", value (0)=w687) -> (output string=w693:string)
                n327 = xnode "Match Regular Expression"("input string"=w688, "regular expression"="((_[0-9]+)?)(\\..[^.]*$)") -> ("before match"=w695:string, "submatch 3"=w690:string)  [unwired: 4 in, 6 out]
                n328 = Concatenate Strings "Append depth number"(w695, w693, w690) -> (w689:string)
                n329 = Build Path(base path=w699, name or relative path=w689) -> (appended path=w696:path)
                n330 = Bundle By Name(cluster=T13 {"State"=enum."Open", "Para."=variant}, "Para."=w696) -> (w697:T13)
              }
            }
            n331 = Select(t=T13 {"State"=enum."Close", "Para."=variant}, s=w663, f=w672) -> (s? t:f=w677:T13)
            n332 = Enqueue Element(queue=w670, element=w677) -> ()  [unwired: 2 in, 3 out]
          }
          frame "Close" {
            # "need to reset registers?\n\nNo"
            n333 = Unbundle By Name(w829) -> ("file refnum"=w830:refnum<file>)
            n334 = property on="Cancel" class="Bool"("Visible"=FALSE) -> ()  [unwired: 2 in, 2 out]
            n335 = property on="Close/Quit" class="Bool (strict)"("BoolText.Text"="Done" ("Boolean Text.Text")) -> ()  [unwired: 2 in, 2 out]
            n336 = Close File(refnum=w830, error in=w827) -> (error out=w826:errorcluster)  [unwired: 1 out]
            n337 = call <vilib>:"Clear Errors.vi"("error in (no error)"=w826) -> ()  [unwired: 5 in, 2 out]
            n338 = Unbundle By Name(w837) -> ("ControlRefs.MainDAQCoreQueue"=w823:refnum<queue>, "ControlRefs.ProcCore_CtrlQueue"=w834:refnum<queue>, "ControlRefs.WriterSIG"=w836:refnum<queue>, "ControlRefs.ProcCore_SignalBuffer"=w824:refnum<queue>, "MultiRec Mode"=w825:bool)
            n339 = case shown="False" w825 {
              tunnel: w836 -> [w846 _]
              tunnel: w834 -> [w843 _]
              tunnel: w824 -> [_ w851]
              tunnel: w823 -> [_ w850]
              frame False {
                n340 = Bundle By Name(cluster=T19 {"Command"=enum."SetWriterRef", "Params"=variant} ("element"), "Command"=ProcessStates."StopSave") -> (w842:T19)
                n341 = Bundle By Name(cluster=T19 {"Command"=enum."SetWriterRef", "Params"=variant} ("element"), "Command"=ProcessStates."SetWriterRef", "Params"=w846) -> (w848:T19)
                n342 = Enqueue Element(queue=w843, element=w842) -> (queue out=w841:refnum<queue>, error out=w840:errorcluster)  [unwired: 2 in, 1 out]
                n343 = Enqueue Element(queue=w841, element=w848, error in (no error)=w840) -> (error out=w839:errorcluster)  [unwired: 1 in, 2 out]
                n344 = call <vilib>:"Clear Errors.vi"("error in (no error)"=w839) -> ()  [unwired: 5 in, 2 out]
              }
              frame True {
                n345 = Bundle By Name(cluster=T21 {"GenericDAQ State"=enum."SetDynamicBuffer_", "Variant"=variant} ("element"), "Variant"=w851) -> (w852:T21)
                n346 = Enqueue Element "Set Data queue"(queue=w850, element=w852) -> ()  [unwired: 2 in, 3 out]
              }
            }
          }
          frame "Quit" {
            n347 = Release Queue(queue=w855) -> ()  [unwired: 2 in, 3 out]
            n348 = disable-structure shown="Enabled" {
              disable-tunnel: w860 -> [w876 w877]
              disable-tunnel: w854 -> [w872 _]
              frame Enabled {
                w870 = nan  # Quit
                # "fundamental, any dequeue should be able to handle e-stop"
                # "Bad solution: have upper level jump out wait queue\n\nThe reason of this is to have MotionCtrl part quit waiting for positions. \n\nalternative method could try to release the queue to do that too. (issue with error 0, must be handled)"
                n349 = Unbundle By Name(w872) -> ("File Header.Start Position"=w871:dbl[])
                n350 = Bundle By Name(cluster=T23 {"Line Start"=[], "Line End"=[], "HighSpeed"=0.0, "ScanSpeed"=0.0, "KeepStill(ms)"=0, "SecendaryParams"=variant} ("element"), "HighSpeed"=w870, "ScanSpeed"=w870, "Line Start"=w871) -> (w873:T23)
                n351 = Enqueue Element(queue=w876, element=w873) -> (error out=w874:errorcluster)  [unwired: 2 in, 2 out]
                n352 = call <vilib>:"Clear Errors.vi"("error in (no error)"=w874) -> ()  [unwired: 5 in, 2 out]
              }
              frame Disabled {
                n353 = Release Queue(queue=w877) -> ()  [unwired: 2 in, 3 out]
              }
            }
            n354 = Generate User Event(user event=w865, event data cluster=cluster{bool} {TRUE} ("event data")) -> (user event out=w863:refnum<user-event>, error out=w862:errorcluster)  [unwired: 2 in]
            n355 = Destroy User Event(user event=w863, error in=w862) -> (error out=w861:errorcluster)
            n356 = Merge Errors(w861, w856) -> (w857:errorcluster)
          }
          frame "Refresh_Image" {
            # "Call command has to be push to the end not start of the queue."
            n357 = Unbundle By Name(w892) -> ("Para."=w891:variant)
            n358 = Variant To Data(type=1 ("PeakOI #"), Variant=w891) -> (data=w878:i32)  [unwired: 1 in, 1 out]
            n359 = Array Subset(array=w895, index (dim 2)=w878, length (dim 2)=1 ("length")) -> (w894:dbl[][][])  [unwired: 4 in]
            n360 = control-ref of="ImagePreview"() -> (w884:refnum<vi>)
            n361 = Array Size(array=w894) -> (size(s)=w893:i32[])
            n362 = Index Array(array=w893) -> (element #1=w889:i32, element #2=w888:i32)  [unwired: 3 in, 1 out]
            n363 = Max & Min(x=w889, y=w888) -> (max(x,y)=w887:i32)  [unwired: 1 out]
            n364 = Reshape Array(w894, w889, w888) -> (w880:dbl[][])
            n365 = property on="Fix race condition \n(autoscale related)" class="IntGraph (strict)"(reference=w884, "Value"=w880) -> (reference out=w885:refnum<vi>, error out=w886:errorcluster)  [unwired: 1 in]
            n366 = property class="IntGraph (strict)" props=["ZScale", "Maximum"](reference=w885, error in=w886) -> (reference out=w882:refnum<vi>)  [unwired: 2 out]
            n367 = case shown="True" "AutoScaleZ" {
              tunnel: w880 -> [_ w912]
              tunnel: w882 -> [_ w909]
              frame False {
              }
              frame True {
                w917 = 256.0
                n368 = Unbundle("Contrast") -> (w906:dbl, w908:dbl)
                n369 = Max & Min(x=w906, y=w908) -> (max(x,y)=w907:dbl, min(x,y)=w905:dbl)
                n370 = Array Max & Min(array=w912) -> (max value=w919:dbl, min value=w915:dbl)  [unwired: 2 out]
                n371 = Subtract(x=w919, y=w915) -> (x-y=w913:dbl)
                n372 = Compound Arithmetic op=MULTIPLY(invert w917, w905, w913) -> (w916:dbl)
                n373 = Compound Arithmetic op=MULTIPLY(invert w917, w913, w907) -> (w914:dbl)
                n374 = Add(x=w914, y=w915) -> (x+y=w910:dbl)
                n375 = Add(x=w915, y=w916) -> (x+y=w911:dbl)
                n376 = property class="IntGraph (strict)"(reference=w909, "ZScale.Maximum"=w910, "ZScale.Minimum"=w911) -> ()  [unwired: 1 in, 2 out]
              }
            }
            n377 = case shown="True" "Full Image" {
              tunnel: w887 -> [_ w904]
              tunnel: w882 -> [_ w902]
              frame False {
              }
              frame True {
                w903 = 0.0
                n378 = property class="IntGraph (strict)"(reference=w902, "XScale.Minimum"=w903, "XScale.Maximum"=w904, "YScale.Minimum"=w903, "YScale.Maximum"=w904) -> ()  [unwired: 1 in, 2 out]
              }
            }
          }
          frame "Save_Image" {
            # "Call command has to be push to the end not start of the queue."
            n379 = control-ref of="Peaks of Interest (32 max)"() -> (w930:refnum<vi>)
            n380 = Unbundle By Name(w961) -> ("Para."=w960:variant)
            n381 = property class="Tbl (strict)"(reference=w930) -> ("Value"=w929:string[][])  [unwired: 1 in, 2 out]
            n382 = Variant To Data(type=1 ("PeakOI #"), Variant=w960) -> (data=w928:i32)  [unwired: 1 in, 1 out]
            n383 = Unbundle By Name(w921) -> ("file path"=w920:path)
            n384 = Index Array(array=w929, index (row) #1=w928, index (col) #1=0 ("disabled index (col)"), index (row) #2=w928, index (col) #2=1 ("disabled index (col)")) -> (element #1=w925:string, element #2=w924:string)
            n385 = control-ref of="ImagePreview"() -> (w955:refnum<vi>)
            n386 = Strip Path(path=w920) -> (stripped path=w935:path, name=w939:string)
            n387 = Array Subset(array=w964, index (dim 2)=w928, length (dim 2)=1 ("length")) -> (w963:dbl[][][])  [unwired: 4 in]
            n388 = property class="IntGraph (strict)" props=["Color Table", "ZScale", "Maximum", "ZScale", "Minimum", "XScale", "Minimum", "XScale", "Maximum", "YScale", "Minimum", "YScale", "Maximum"](reference=w955) -> ("Color Table"=w932:u32[], "ZScale.Maximum"=w933:dbl, "ZScale.Minimum"=w934:dbl)  [unwired: 1 in, 6 out]
            n389 = xnode "Match Regular Expression"("input string"=w939, "regular expression"="(\\..[^.]*$)") -> ("before match"=w952:string)  [unwired: 4 in, 4 out]
            n390 = Format Into String(format string="_%s(+-%s)", w925, w924) -> (resulting string=w951:string)  [unwired: 2 in, 1 out]
            n391 = Array Size(array=w963) -> (size(s)=w962:i32[])
            n392 = Index Array(array=w962) -> (element #1=w957:i32, element #2=w956:i32)  [unwired: 3 in, 1 out]
            n393 = Concatenate Strings(w952, w951, ".png" ("string")) -> (w936:string)
            n394 = Reshape Array(w963, w957, w956) -> (w931:dbl[][])
            n395 = Subtract(x=w933, y=w934) -> (x-y=w945:dbl)
            n396 = Build Path(base path=w935, name or relative path=w936) -> (appended path=w937:path)
            n397 = Subtract(x=w931, y=w934) -> (x-y=w954:dbl[][])
            n398 = Divide(x=256.0 ("Img_coeff."), y=w945) -> (x/y=w947:dbl)
            n399 = Array Size(array=w954) -> (size(s)=w940:i32[])
            n400 = Compound Arithmetic op=MULTIPLY(w947, w954) -> (w948:dbl[][])
            n401 = Transpose 2D Array(2D array=w948) -> (transposed array=w949:dbl[][])
            n402 = Index Array(array=w940) -> (element #1=w942:i32, element #2=w943:i32)  [unwired: 2 in]
            n403 = Round Toward -Infinity(1:w949) -> (0:w950:dbl[][])
            n404 = Multiply(x=w942, y=w943) -> (x*y=w944:i32)
            n405 = To Unsigned Byte Integer(number=w950) -> (unsigned 8bit integer=w941:u8[][])
            n406 = disable-structure shown="Enabled" {
              disable-tunnel: w932 -> [w980 _]
              disable-tunnel: w937 -> [w979 w983]
              disable-tunnel: w941 -> [w975 w984]
              disable-tunnel: w942 -> [w973 _]
              disable-tunnel: w943 -> [w972 _]
              disable-tunnel: w944 -> [w971 _]
              frame Enabled {
                n407 = Reshape Array(w975, w971) -> (w974:u8[])
                n408 = Bundle By Name(cluster=T24 {"image type"=0, "image depth"=32, "image"=[], "mask"=[], "colors"=[], "Rectangle"={"left"=0, "top"=0, "right"=256, "bottom"=256}} ("Image Data 2"), "colors"=w980, "image type"=0, "image depth"=8, "image"=w974, "Rectangle.right"=w973, "Rectangle.bottom"=w972) -> (w970:T24)
                n409 = call <vilib>:"Write PNG File.vi"("image data"=w970, "path to PNG file"=w979) -> ("error out"=w969:errorcluster)  [unwired: 8 in, 1 out]
                n410 = call <vilib>:"Clear Errors.vi"("error in (no error)"=w969) -> ()  [unwired: 5 in, 2 out]
              }
              frame Disabled {
                n411 = call "IMAQ ArrayToImage"("Image Pixels (U8)"=w984) -> ("Image Out"=w982:T27)  [unwired: 9 in, 1 out]
                n412 = call-poly "IMAQ Write File 2"("TIFF Options"=T25 {"Rows Per Strip"=0, "Photometric"=1, "Compression Type"=3}, "File Path"=w983, "Image"=w982) -> ()  [unwired: 7 in, 2 out]
              }
            }
          }
          frame "SetPeakOI" {
            n413 = Unbundle By Name(w1103) -> ("PeakOI"=w1099:cluster{"m/z":dbl, "Width(+/-)":dbl}[])
            n414 = Unbundle By Name(w1105) -> ("Para."=w1104:variant)
            n415 = Variant To Data(type=w1099, Variant=w1104) -> (data=w1101:cluster{"m/z":dbl, "Width(+/-)":dbl}[], error out=w1102:errorcluster)  [unwired: 1 in]
            n416 = Select(t=w1099, s=w1102, f=w1101) -> (s? t:f=w1100:cluster{"m/z":dbl, "Width(+/-)":dbl}[])
            n417 = Bundle By Name(cluster=w1103, "PeakOI"=w1100) -> (w1108:T8)
          }
          frame Default {
          }
        }
        n418 = call <userlib>:"ErrorLog.vi"("error in (no error)"=w227) -> ("error out"=w226:errorcluster)  [unwired: 10 in]
      }
      frame Error {
      }
    }
    "Iteration" <- w202
  }
  n419 = while {
    tunnel: w4 -> [w1130]
    stop <- w1129 stop-if-true
    n420 = Get Queue Status(queue=w1130, return elements? (F)=TRUE) -> (error out=w1129:errorcluster, elements=w1126:i32[])  [unwired: 1 in, 6 out]
    n421 = Reverse 1D Array(array=w1126) -> (reversed array=→"elements":i32[])
    n422 = Wait Until Next ms Multiple(millisecond multiple=u32 1000) -> ()  [unwired: 1 out]
  }
  n423 = disable-structure shown="Disabled" {
    frame Disabled {
      n424 = Unbundle By Name() -> ("Binning.Maximum"=w1131:dbl, "Binning.BinWidth"=w1132:dbl, "Binning.Enable"=w1136:bool, "Binning.Minimum"=w1133:dbl, "m/z_Array"=w1135:dbl[], "Binning.BinType"=w1134:T11)  [unwired: 1 in]
      n425 = case "Batch Binning" shown="True" w1136 {
        selector: w1136 -> [_ w1142]
        tunnel: w1131 -> [_ w1147]
        tunnel: w1132 -> [_ w1146]
        tunnel: w1133 -> [_ w1145]
        tunnel: w1134 -> [_ w1144]
        tunnel: w1135 -> [w1138 w1143]
        tunnel: [w1139 w1141] -> w1137
        frame False {
          n426 = Array Size(array=w1138) -> (size(s)=w1139:i32)
        }
        frame True {
          n427 = call "SpectrumBinning_NoGraph.vi"("XScale.Maximum"=w1147, "BinType"=w1144, "BinWidth"=w1146, "Enable"=w1142, "m/z Array"=w1143, "XScale.Minimum"=w1145) -> ("m/z Array"=w1140:dbl[])  [unwired: 3 in, 2 out]
          n428 = Array Size(array=w1140) -> (size(s)=w1141:i32)
        }
      }
      n429 = Bundle By Name("SpecLength"=w1137) -> ()  [unwired: 1 in, 1 out]
    }
    frame Enabled {
    }
  }
  n430 = Release Queue "Release Queue\nAfter all quit."(queue=w33, error in (no error)=w35) -> (error out=→"error out":errorcluster)  [unwired: 1 in, 2 out]
